vi "Turbulence_3.1_FullAuto.vi"() -> ()   [LabVIEW 2018]
uses:
  <instrlib>/Quantum Composers 9000 Series 2.08/Quantum Composers 9000 Series.lvlib
  <userlib>/LightField Add-in and Automation SDK/Samples/LabVIEW Automation/lightfield-automation-labview/LightField Automation.lvclass
  <instrlib>/Mercury iXX/Mercury iXX.lvlib
  <instrlib>/Mercury iXX/Public/Libraries/Temperature/Signals/Read/Temperature (Read).vi
  <instrlib>/Mercury iXX/Public/Libraries/Temperature.lvlib
  <instrlib>/Mercury iXX/Public/Libraries/Temperature/Open/Open Temperature Device.vi
  <instrlib>/Mercury iXX/Public/Controls/Comms Transport Layer.ctl
  <instrlib>/Keithley 2600 Series/Keithley 2600 Series.lvlib
  <instrlib>/Keithley 2600 Series/Public/Channel.ctl
  <vilib>/DAQmx/read.llb/DAQmx Read (Counter DBL 1Chan 1Samp).vi
  <instrlib>/Mercury iXX/Public/Libraries/System/Read/Catalogue (Read).vi
  <instrlib>/Mercury iXX/Public/Libraries/System.lvlib
  <instrlib>/Mercury iXX/Public/Libraries/System/Open/Open System.vi
panel:
  in  "Extra Waits":i32
  in  "Error":bool
  in  "3He Check":bool
  out "MFC Error Out":errorcluster
  out "Lakeshore218 Error":errorcluster
  in  "File Exists":bool
  out "Log":refnum<file>
  in  "Motor free":bool
  in  "RESTART":bool
  out "time string":string
  out "Timestamp":string
  out "Log Error":errorcluster
  in  "CLOSE":bool
  in  "RECORD":bool
  in  "Turbulence":T1(tab)
  in  "FROM FILE":bool
  in  "Script File":path
  in  "# Frames":i32=1000 min=0 step=1
  in  "New Background Movie":bool
  in  "On CCD Acc.":i32=3 min=0 step=1
  in  "Cycle time\n(ms)":i32=3 min=0 step=1
  out "High Level\n(Ohms)":dbl format="%.1f"
  out "Low Level\n(Ohms)":dbl format="%.1f"
  in  "New Background Frame":bool
  out "Rate (Hz)":dbl
  out "Incident":dbl
  in  "BIN":u16(ring)=2 items=["1x1", "2x2", "4x4"]
  in  "MODE":u16(ring) items=["Normal", "DIF"]
  in  "Enable":bool
  out "Rate (Hz)":dbl
  out "Detected":dbl
  in  "Script\nEnd":u32=1 step=1
  in  "Sample Space Pump":bool
  in  "Siphon Pump":bool
  in  "Neutron Shutter":bool
  in  "Manual Script Entry (0)":string
  in  "READY":bool
  out "Power (mW)":dbl format="%_3f"
  out "Tank Pressure 2 (Torr)":string="0.0"
  in  "LIGHTFIELD":bool
  in  "SCRIPTING":bool
  in  "Top Coil":bool
  out "Tank Pressure 1 (Torr)":string="0.0"
  out "Cell (K)":dbl format="%.3f"
  out "Cryostat (K)":dbl format="%.3f"
  in  "Data Interval (s)":dbl=0.5 min=0.4 max=10.0 step=0.05
  in  "RUN/STOP":bool
  in  "Bottom Coil":bool
  in  "Bottom Coil (mA)":dbl min=-1000.0 max=1000.0 step=1e-05
  in  "Top Coil (mA)":dbl min=-1000.0 max=1000.0 step=1e-05
  in  "Percent Open":i32 min=0 max=100 step=5
  in  "COOLDOWN":bool
  in  "Script\n#":i32 step=1
  in  "Kill Switch":bool
  in  "DATA":bool
  out "Scripting Error":T2
  in  "Shutter Mode":u16(ring)=1 items=["Manual"=1, "XGate"=5]
  in  "Time (s)":i32=120 min=1 max=300 step=1
  in  "REFILL":bool
  in  "AUTOFILL":bool
  in  "LL (Ohms)":dbl=900.0 min=750.0 max=15000.0 step=1.0
  in  "HL (Ohms)":dbl=900.0 min=750.0 max=15000.0 step=1.0
  in  "Fill":bool
  in  "Tare":bool
  out "Actual 3He\nTank Pressure":dbl min=0.0 max=100.0 step=5.0 format="%#.1g"
  out "Desired V2\nPressure (3He)":dbl min=0.0 max=100.0 step=5.0 format="%#.1f"
  in  "Desired Tank\nPressure (3He)":dbl min=0.0 max=100.0 step=0.01 format="%#.2f"
  in  "Log Pressure":bool
  out "4He Pressure (Torr)":string="-0.1"
  out "3He Pressure (Torr)":string="1"
  in  "Fill Time (s)":u32=10
  out "Temperature Error":errorcluster={"status"=TRUE, "code"=-1073807339, "source"="VISA Read in Mercury iXX.lvlib:Query (Dynamic).vit->Mercury iXX.lvlib:Query (Low Level).vi:10049->Mercury iXX.lvlib:Query.vi:3960048->Mercury iXX.lvlib:Read (Str).vi:5300004->Mercury iXX.lvlib:System.lvlib:Catalogue (Read).vi->Turbulence.vi"}
  out "File I/O Error":errorcluster
  out "4He Gauge Error":errorcluster={"status"=TRUE, "code"=-1073807343, "source"="VISA Open in Turbulence.vi"}
  out "Heater Error":errorcluster={"status"=FALSE, "code"=1073676293, "source"="VISA Read in Keithley 2600 Series.lvlib:Print Number.vi->Keithley 2600 Series.lvlib:Measure.vi->Turbulence.vi"}
  out "Pulse Generator Error":errorcluster
  out "3He Gauge Error":errorcluster={"status"=FALSE, "code"=1073676293, "source"="VISA Read in 3HeClose.vi->Turbulence.vi"}
  out "Relay Errror":errorcluster
  out "Zaber Motor Error":errorcluster
  out "LightField Error":errorcluster
  out "Shutter Error":errorcluster
  # "Camera Controls"
  # "Temperature Readout"
  # "Pressure Readout"
  # "Neutron Counts"
  # "Automation"
  # "Heater Controls"
  # "Relay Controls"
  # "Needle Valve Control"
  # "Neutron Shutter"
  # "Optical Shutter"
  # "Siphon Pump"
  # "Laser Power Meter"
  # "Sample Space\nPump"
  # "V1 = 4075 mL"
  # "V2 = 15.5 mL"
  # "V3 = 78.8 mL"
  # "Quartz\nCell"
  # "4"
  # "3psi relief"
  # "MFC"
  # "V1"
  # "4L Tank"
  # "Turbo Pump"
  # "V2"
  # "V3"
  # "3"
  # "10psi relief"
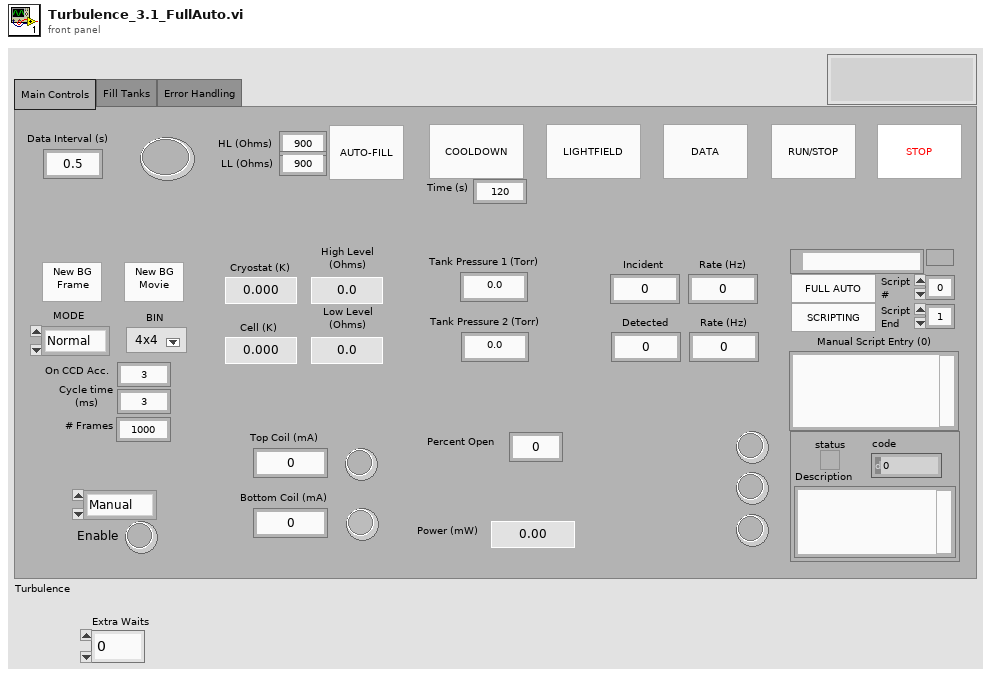
[diagram p1: front panel]
types:
  T1 = enum32{"Main Controls", "Fill Tanks", "Error Handling"}
  T2 = cluster{"status":bool, "code":i32, "Description":string}
  T3 = typedef "Mercury iXX.lvlib/Comms Transport Layer.ctl" = enum16{"Ethernet TCP/IP", "USB", "ISOBus - RS-232", "GPIB"}
  T4 = typedef "Mercury iXX.lvlib/Mercury Reference.ctl" = cluster{"Comms":refnum<visa-resource-name>, "Device ID":string[], "Comms Layer":T3, "Command":string, "Query reference":T5}
  T5 = typedef "Mercury iXX.lvlib/Query Dynamic Reference.ctl" = refnum<vi>
  T6 = enum32{"Current", "Voltage", "IV", "Resistance", "Power"}
  T7 = typedef "Keithley 2600 Series.lvlib/Channel.ctl" = enum32{"Channel A", "Channel B"}
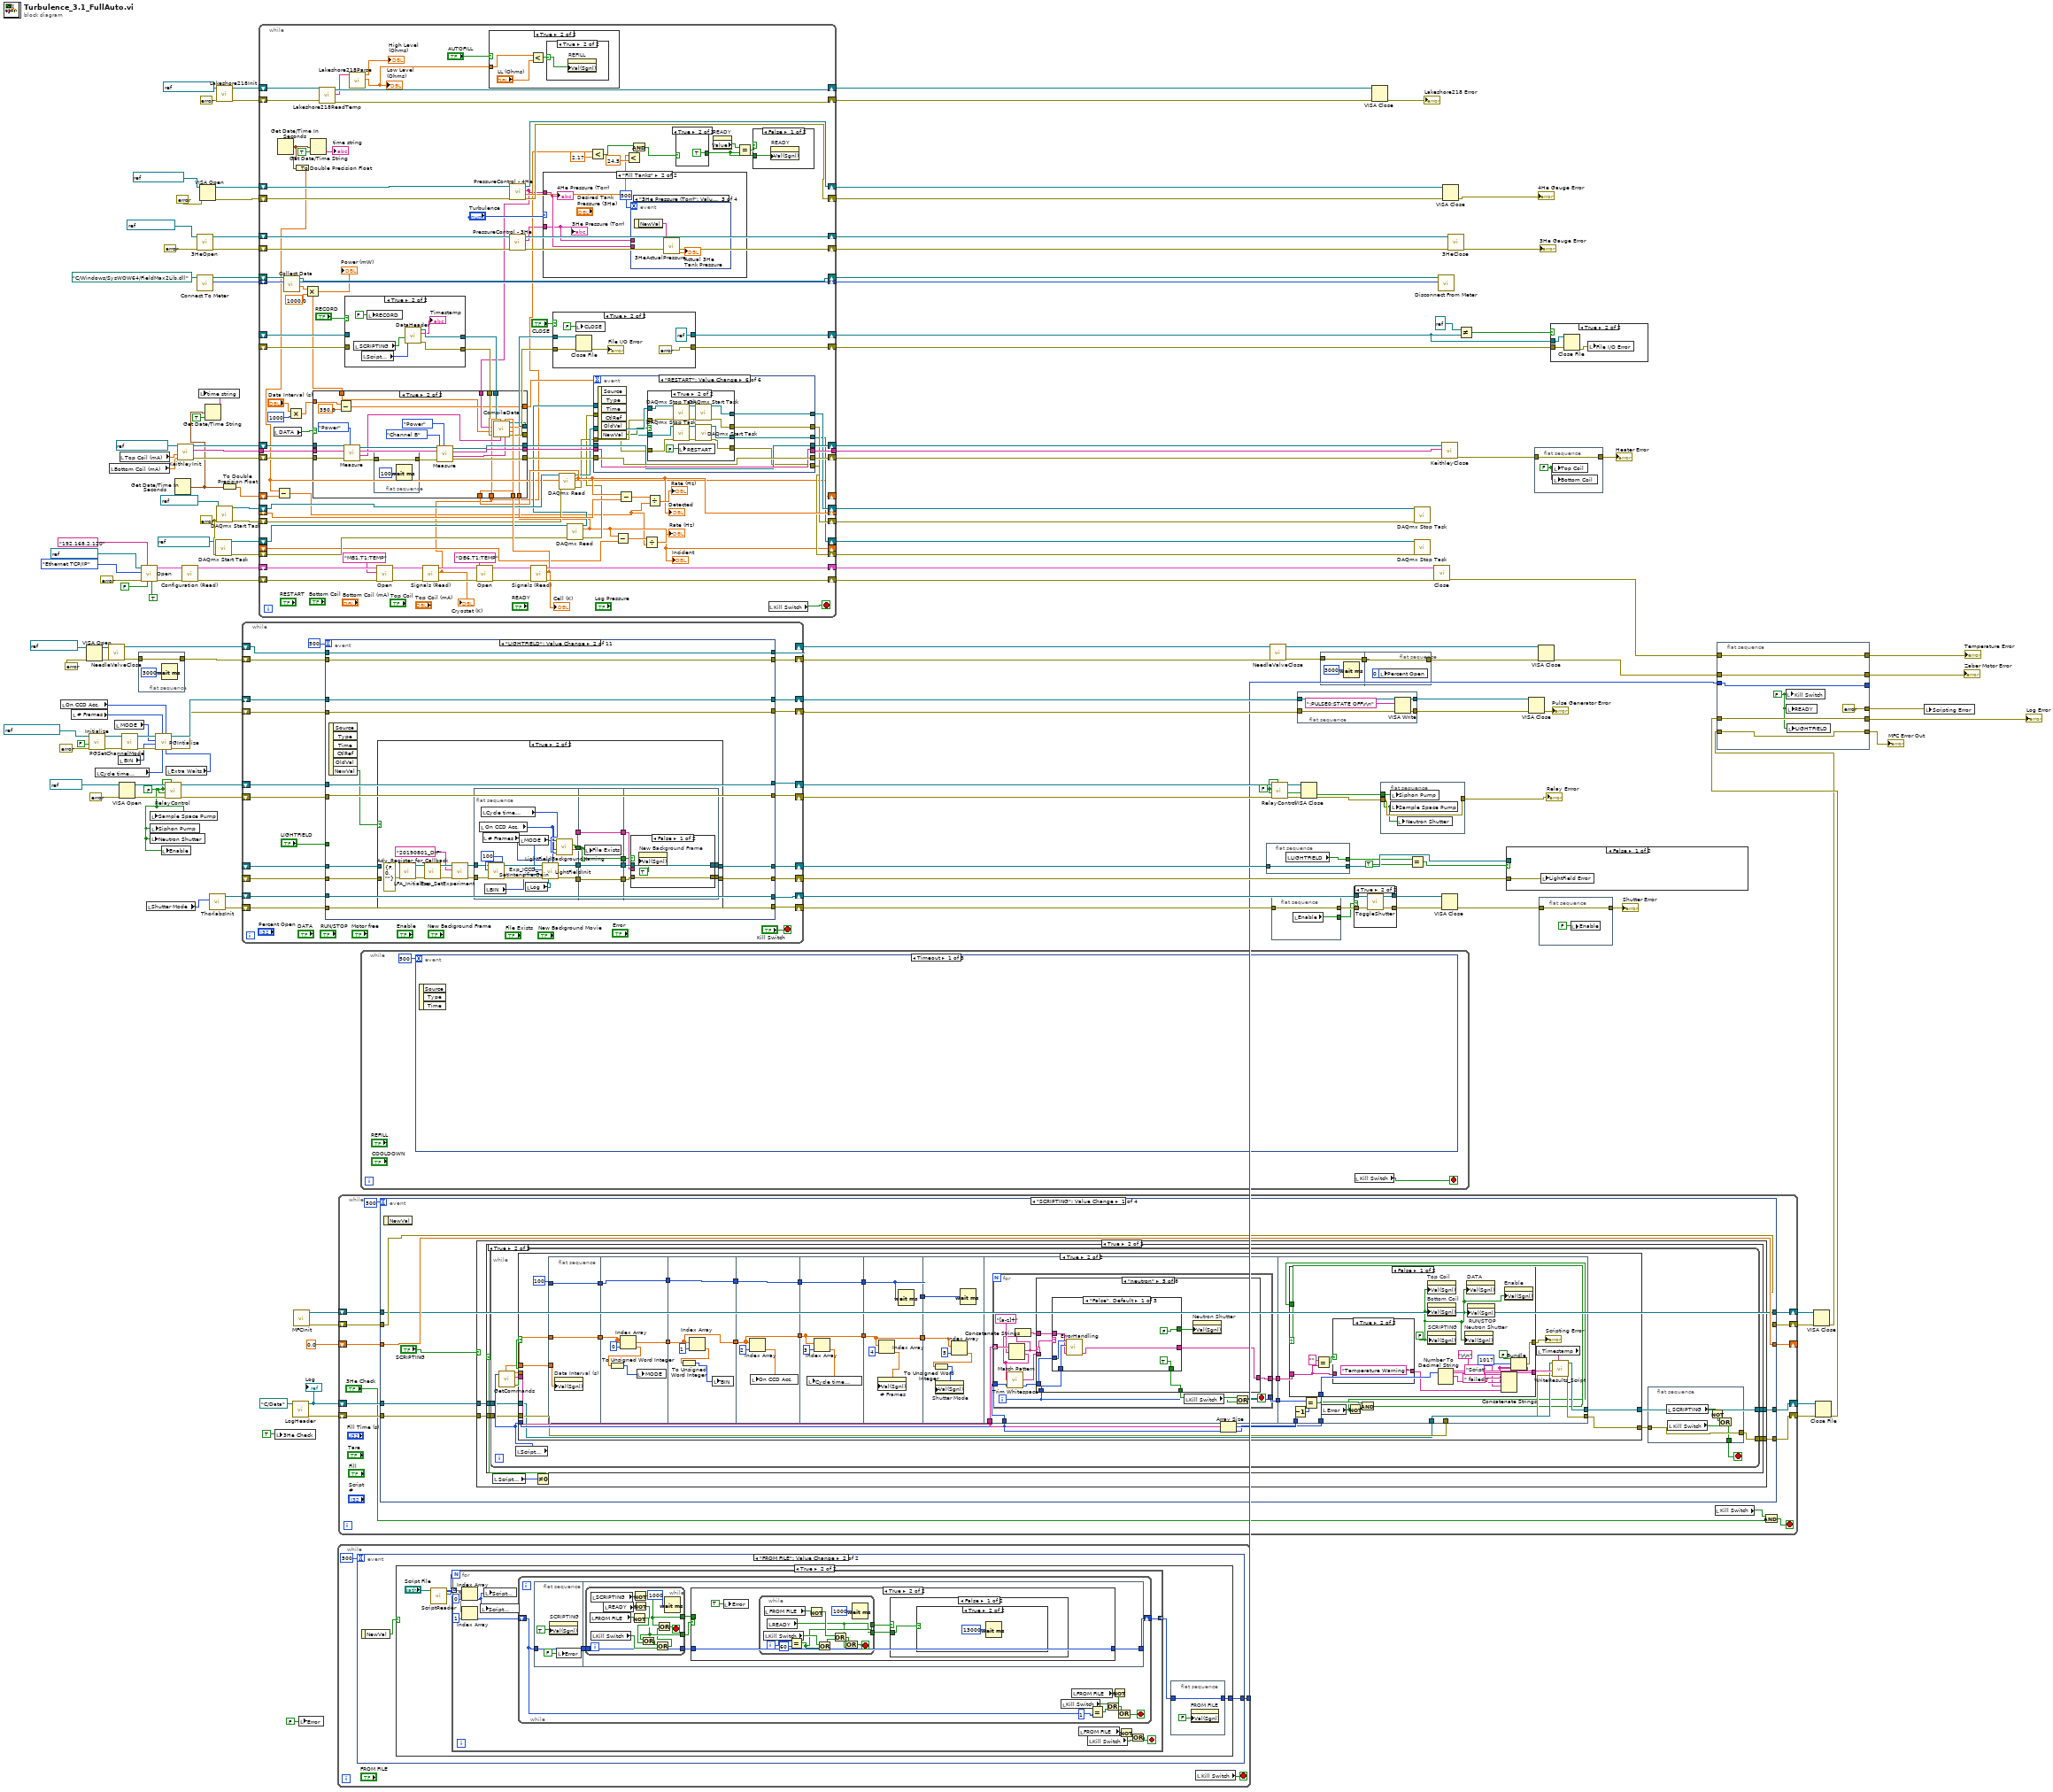
[diagram p0: block diagram]
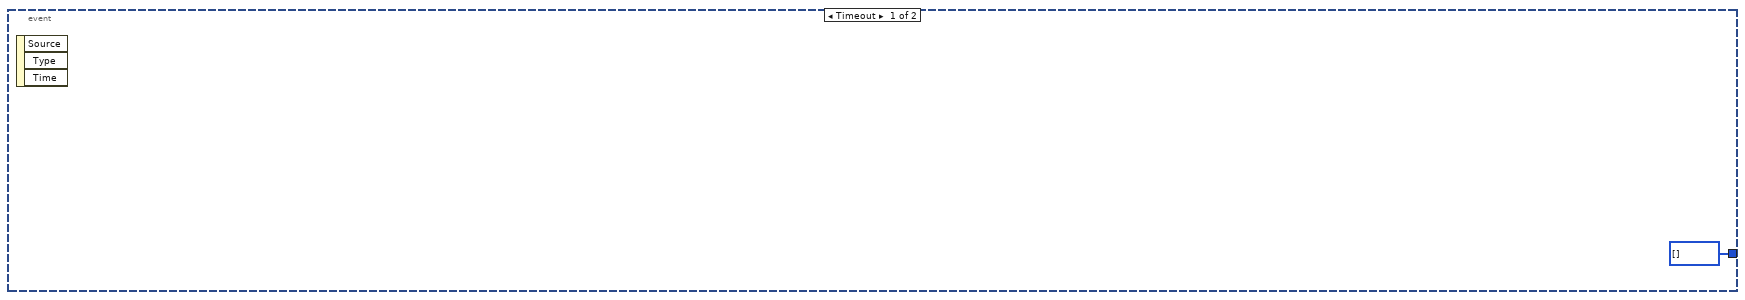
[diagram p2: hidden frame]
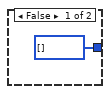
[diagram p3: hidden frame]
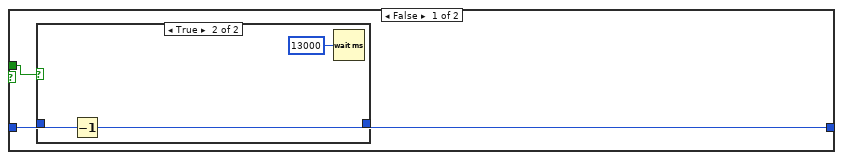
[diagram p4: hidden frame]
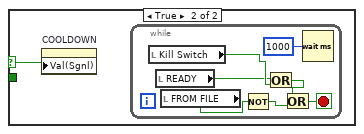
[diagram p7: hidden frame]
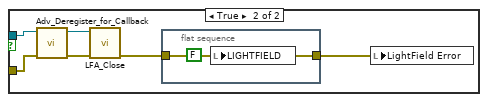
[diagram p9: hidden frame]
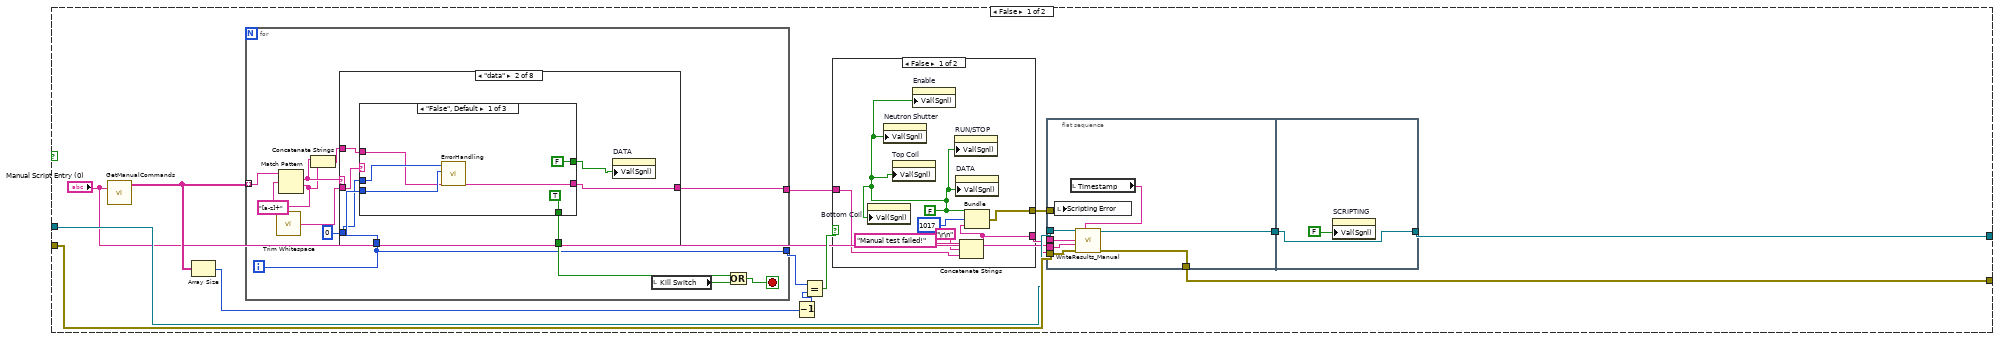
[diagram p11: hidden frame]
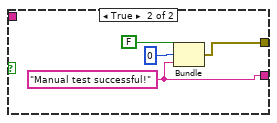
[diagram p12: hidden frame]
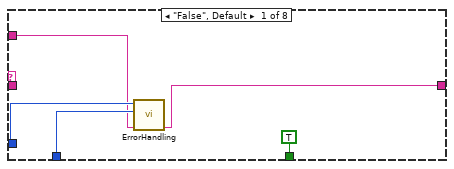
[diagram p13: hidden frame]
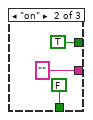
[diagram p14: hidden frame]
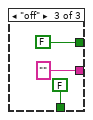
[diagram p15: hidden frame]
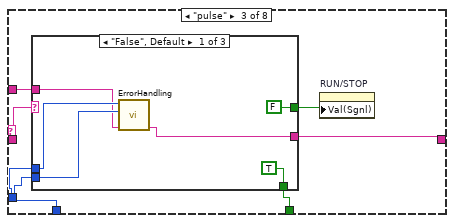
[diagram p16: hidden frame]
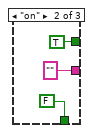
[diagram p17: hidden frame]
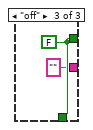
[diagram p18: hidden frame]
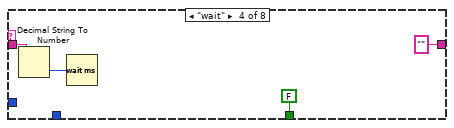
[diagram p19: hidden frame]
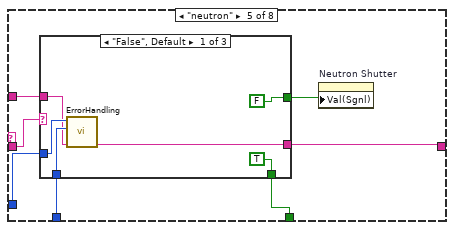
[diagram p20: hidden frame]
diagram:
  w42 = errorcluster {"status"=FALSE, "code"=0, "source"=""} ("error in")
  w79 = FALSE ("Siphon Pump")
  w64 = FALSE ("Siphon Pump")
  n1 = local read "On CCD Acc."() -> (w53:i32)
  n2 = local read "# Frames"() -> (w52:i32)
  n3 = VISA Open(error in (no error)=errorcluster {"status"=FALSE, "code"=0, "source"=""}, VISA resource name=refnum<visa-resource-name> "ZaberMotor") -> (VISA resource name=w59:refnum<visa-resource-name>, error out=w60:errorcluster)  [unwired: 3 in]
  n4 = call <instrlib>:"Initialize.vi"("error in (no error)"=errorcluster {"status"=FALSE, "code"=0, "source"=""}, "Reset? (T: Yes)"=FALSE, "VISA resource name"=refnum<visa-resource-name> "PulseGenerator" ("Pulse generater (COM3)")) -> ("error out"=w71:errorcluster, "VISA resource name out"=w69:refnum<visa-resource-name>)  [unwired: 7 in]
  n5 = local read "Cycle time\n(ms)"() -> (w13:i32)
  n6 = call "NeedleValveClose.vi"("error in (no error)"=w60, "VISA resource name"=w59) -> ("error out"=w61:errorcluster, "VISA resource name out"=w101:refnum<visa-resource-name>)  [unwired: 8 in]
  n7 = local read "Bottom Coil (mA)"() -> (w113:dbl)
  n8 = local read "MODE"() -> (w50:u16)
  n9 = local read "BIN"() -> (w51:u16)
  n10 = VISA Open(error in (no error)=errorcluster {"status"=FALSE, "code"=0, "source"=""} ("error in (no error) 2"), VISA resource name=refnum<visa-resource-name> "Relays" ("Pressure Gauge")) -> (VISA resource name=w126:refnum<visa-resource-name>, error out=w128:errorcluster)  [unwired: 3 in]
  n11 = local read "Top Coil (mA)"() -> (w114:dbl)
  n12 = call "PGSetChannelMode.vi"("error in"=w71, "VISA resource name"=w69) -> ("error out"=w70:errorcluster, "VISA resource name out"=w68:refnum<visa-resource-name>)  [unwired: 8 in]
  n13 = flat-sequence {
    tunnel: w61 -> [w155]
    tunnel: [w155] -> w102
    frame #0 {
      n14 = Wait (ms)(milliseconds to wait=u32 3000) -> ()  [unwired: 1 out]
    }
  }
  n15 = call-poly <instrlib>:"Open.vi"("Clear Previous Connections (False)"=TRUE, "ID Query (True)"=FALSE, "IP Address"="192.168.2.120", "error in (no error)"=errorcluster {"status"=FALSE, "code"=0, "source"=""}, "Comms Layer"=Comms_Transport_Layer."Ethernet TCP/IP", "VISA resource name"=refnum<visa-resource-name> "MercuryiTC") -> ("error out"=w147:errorcluster, "Mercury Reference Out"=w148:T4)  [unwired: 1 in, 3 out]
  n16 = local read "Shutter Mode"() -> (w54:u16)
  n17 = local write "Sample Space Pump"(w64) -> ()
  n18 = local write "Neutron Shutter"(w64) -> ()
  n19 = local write "Siphon Pump"(w64) -> ()
  n20 = local write "Enable"(w64) -> ()
  n21 = call "RelayControl.vi"("Neutron Shutter"=w64, "Error In"=w128, "Sample Space Pump"=w64, "Siphon Pump"=w64, "Relay In"=w126) -> ("Error Out"=w127:errorcluster, "Relay Out"=w125:refnum<visa-resource-name>)  [unwired: 5 in]
  n22 = local read "Extra Waits"() -> (w1:i32)
  n23 = call "PGIntialize.vi"("Extra Waits"=w1, "On CCD Accumulations"=w53, "Cycle time\n(ms)"=w13, "Number of Frames"=w52, "error in"=w70, "BIN"=w51, "MODE"=w50, "VISA resource name"=w68) -> ("error out"=w152:errorcluster, "VISA resource name out"=w153:refnum<visa-resource-name>)  [unwired: 2 in]
  n24 = Get Date/Time In Seconds() -> (seconds since 1Jan1904=w21:timestamp)
  n25 = call "KeithleyInit.vi"("Bottom Coil (mA)"=w113, "Top Coil (mA)"=w114, "KeithleyVISA In"=refnum<visa-resource-name> "Keithley2614B" ("VISA resource name")) -> ("error out"=w117:errorcluster, "Node Out"=w118:string, "KeithleyVISA Out"=w116:refnum<visa-resource-name>)  [unwired: 6 in]
  n26 = call-poly <instrlib>:"Configuration (Read).vi"("error in"=w147, "Mercury Reference In"=w148) -> ("error out"=w143:errorcluster, "Mercury Reference Out"=w144:T4)  [unwired: 6 in, 2 out]
  n27 = call "Connect To Meter.vi"("Location of FieldMax2Lib.dll in"=path "C:/Windows/SysWOW64/FieldMax2Lib.dll") -> ("Meter ID out"=w87:i32, "Location of FieldMax2Lib.dll out"=w86:path)  [unwired: 6 in, 1 out]
  n28 = call "3HeOpen.vi"("error in (no error)"=errorcluster {"status"=FALSE, "code"=0, "source"=""} ("error in (no error) 2"), "VISA resource name"=refnum<visa-resource-name> "3HePressure" ("Pressure Gauge")) -> ("error out"=w130:errorcluster, "VISA resource name out"=w129:refnum<visa-resource-name>)  [unwired: 8 in]
  n29 = VISA Open(error in (no error)=errorcluster {"status"=FALSE, "code"=0, "source"=""} ("error in (no error) 2"), VISA resource name=refnum<visa-resource-name> "TankPressure" ("Pressure Gauge")) -> (VISA resource name=w140:refnum<visa-resource-name>, error out=w141:errorcluster)  [unwired: 3 in]
  n30 = Get Date/Time String(seconds (now)=w21, want seconds? (F)=TRUE) -> (time string=w22:string)  [unwired: 1 in, 1 out]
  n31 = local write "time string"(w22) -> ()
  n32 = call "ThorlabsInit.vi"("Shutter Mode"=w54) -> ("error out"=w65:errorcluster, "VISA resource name out"=w66:refnum<visa-resource-name>)  [unwired: 9 in]
  n33 = call <vilib>:"DAQmx Start Task.vi"("task/channels in"=refnum<k21> "IncidentBeam", "error in"=w42) -> ("task out"=w44:refnum<k21>, "error out"=w43:errorcluster)  [unwired: 12 in]
  n34 = call "Lakeshore218Init.vi"("error in (no error)"=errorcluster {"status"=FALSE, "code"=0, "source"=""}, "VISA resource name"=refnum<visa-resource-name> "Lakeshore218") -> ("error out"=w19:errorcluster, "VISA resource name out"=w18:refnum<visa-resource-name>)  [unwired: 8 in]
  n35 = call <vilib>:"DAQmx Start Task.vi"("task/channels in"=refnum<k21> "Detector", "error in"=w42) -> ("task out"=w47:refnum<k21>, "error out"=w46:errorcluster)  [unwired: 12 in]
  n36 = To Double Precision Float(number=w21) -> (double precision float=w24:dbl)
  n37 = while {
    shift-right: [w178] -> w31
    shift-left: _ -> [w176]
    shift-right: [w179] -> w38
    shift-left: _ -> [w177]
    shift-right: [w172] -> w95
    shift-left: w153 -> [w174]
    shift-right: [w173] -> w96
    shift-left: w152 -> [w175]
    shift-right: [w168] -> w100
    shift-left: w127 -> [w171]
    shift-right: [w169] -> w98
    shift-left: w125 -> [w170]
    shift-right: [w163] -> w131
    shift-left: w102 -> [w166]
    shift-right: [w164] -> w132
    shift-left: w101 -> [w165]
    shift-right: [w160] -> w34
    shift-left: w66 -> [w157]
    shift-right: [w159] -> w27
    shift-left: w65 -> [w158]
    stop <- "Kill Switch" stop-if-true
    n38 = event shown="[1] \"LIGHTFIELD\": Value Change" {
      selector: _ -> [_ _ _ _ _ _ _ _ _ _ _]
      dyn-events: _ -> [_ _ _ _ _ _ _ _ _ _ _]
      timeout: 500 -> [_ _ _ _ _ _ _ _ _ _ _]
      tunnel: w175 -> [w187 w196 w273 w319 w337 w386 w451 w470 w485 w508 w533]
      tunnel: w174 -> [w186 w195 w274 w320 w336 w387 w452 w469 w484 w507 w534]
      tunnel: w177 -> [w188 w199 w264 w311 w339 w390 w449 w473 w489 w499 w529]
      tunnel: w176 -> [w189 w200 w265 w312 w340 w391 w450 w474 w488 w500 w530]
      tunnel: [w188 w201 w263 w311 w339 w378 w449 w473 w489 w499 w529] -> w179
      tunnel: [w189 w202 w262 w312 w340 w370 w450 w474 w488 w500 w530] -> w178
      tunnel: [w187 w196 w276 w319 w337 w376 w451 w470 w485 w505 w533] -> w173
      tunnel: [w186 w195 w275 w320 w336 w383 w452 w469 w484 w506 w534] -> w172
      tunnel: w171 -> [w184 w197 w270 w317 w342 w385 w458 w472 w487 w501 w531]
      tunnel: w170 -> [w185 w198 w271 w318 w341 w384 w457 w471 w486 w502 w532]
      tunnel: [w185 w198 w271 w318 w341 w384 w454 w471 w486 w502 w532] -> w169
      tunnel: [w184 w197 w270 w317 w342 w385 w453 w472 w487 w501 w531] -> w168
      tunnel: w166 -> [w183 w194 w269 w321 w325 w389 w448 w468 w483 w503 w535]
      tunnel: w165 -> [w182 w193 w268 w322 w338 w388 w447 w467 w482 w504 w536]
      tunnel: [w182 w193 w268 w322 w335 w388 w447 w467 w482 w504 w536] -> w164
      tunnel: [w183 w194 w269 w321 w327 w389 w448 w468 w483 w503 w535] -> w163
      tunnel: "LIGHTFIELD" -> [_ _ w261 w316 _ w372 _ _ _ w495 _]
      tunnel: w157 -> [w180 w191 w267 w314 w333 w382 w445 w466 w493 w498 w528]
      tunnel: w158 -> [w181 w190 w266 w313 w332 w381 w444 w465 w492 w497 w527]
      tunnel: [w180 w191 w267 w314 w333 w382 w445 w463 w490 w498 w528] -> w160
      tunnel: [w181 w190 w266 w313 w332 w381 w444 w464 w491 w497 w527] -> w159
      event Timeout {
        n39 = event-data() -> ()  [unwired: 1 in, 3 out]
      }
      event "LIGHTFIELD": Value Change {
        n40 = event-data() -> ("NewVal"=w192:bool)  [unwired: 1 in, 5 out]
        n41 = case shown="True" w192 {
          tunnel: [refnum<class "LightField Automation.lvclass"> refnum ("LightField Automation out") w218] -> w202
          tunnel: [errorcluster {"status"=FALSE, "code"=0, "source"=""} ("error out") w217] -> w201
          tunnel: w200 -> [w206 _]
          tunnel: w199 -> [w205 _]
          frame False {
            n42 = call <userlib>:"Adv_Deregister_for_Callback.vi"("error in (no error)"=w205, "LightField Automation in"=w206) -> ("error out"=w208:errorcluster, "LightField Automation out"=w209:refnum<class "LightField Automation.lvclass">)  [unwired: 8 in]
            n43 = call <userlib>:"LFA_Close.vi"("error in (no error)"=w208, "LightField Automation in"=w209) -> ("error out"=→"LightField Error":errorcluster)  [unwired: 8 in, 1 out]
          }
          frame True {
            n44 = call <userlib>:"LFA_Initialize.vi"("error in (no error)"=errorcluster {"status"=FALSE, "code"=0, "source"=""}) -> ("error out"=w227:errorcluster, "LightField Automation out"=w226:refnum<class "LightField Automation.lvclass">)  [unwired: 9 in]
            n45 = call <userlib>:"Adv_Register_for_Callback.vi"("error in (no error)"=w227, "LightField Automation in"=w226) -> ("error out"=w225:errorcluster, "LightField Automation out"=w224:refnum<class "LightField Automation.lvclass">)  [unwired: 8 in]
            n46 = call <userlib>:"Exp_SetExperiment.vi"("error in (no error)"=w225, "ExperimentName"="20190801_DIF", "LightField Automation in"=w224) -> ("error out"=w211:errorcluster, "LightField Automation out"=w210:refnum<class "LightField Automation.lvclass">)  [unwired: 7 in]
            n47 = flat-sequence {
              tunnel: [w238] -> w215
              tunnel: [w236] -> w214
              tunnel: [w235] -> w213
              tunnel: [w239] -> w212
              tunnel: w211 -> [w242]
              tunnel: w210 -> [w240]
              tunnel: [w246] -> w221
              tunnel: [w245] -> w220
              tunnel: [w244] -> w219
              tunnel: [w243] -> w216
              tunnel: w215 -> [w243]
              tunnel: w214 -> [w246]
              tunnel: w213 -> [w245]
              tunnel: w212 -> [w244]
              tunnel: w221 -> [w251]
              tunnel: w220 -> [w252]
              tunnel: w219 -> [w250]
              tunnel: [w249] -> w218
              tunnel: [w248] -> w217
              tunnel: w216 -> [w247]
              frame #0 {
                n48 = local read "On CCD Acc."() -> (w228:i32)
                n49 = local read "Cycle time\n(ms)"() -> (w237:i32)
                n50 = local read "# Frames"() -> (w229:i32)
                n51 = local read "BIN"() -> (w231:u16)
                n52 = call <userlib>:"Exp_ICCD_SetIntensifierGain.vi"("error in (no error)"=w242, "Intensifier Gain"=100, "LightField Automation in"=w240) -> ("error out"=w233:errorcluster, "LightField Automation out"=w234:refnum<class "LightField Automation.lvclass">)  [unwired: 7 in]
                n53 = local read "MODE"() -> (w230:u16)
                n54 = local read "Log"() -> (w232:refnum<file>)
                n55 = call "LightFieldInit.vi"("On CCD Accumulations"=w228, "File Path"=w232, "Number of Frames"=w229, "error in"=w233, "BIN"=w231, "MODE"=w230, "LightField Automation in"=w234) -> ("error out"=w236:errorcluster, "LightField Automation out"=w235:refnum<class "LightField Automation.lvclass">)  [unwired: 3 in]
                n56 = call "LightFieldBackgroundNaming.vi"("Cycle time\n(ms)"=w237, "On CCD Acc."=w228, "MODE"=w230) -> ("FilePath"=w239:string, "Exists"=w238:bool)  [unwired: 6 in, 1 out]
              }
              frame #1 {
                n57 = local write "File Exists"(w243) -> ()
              }
              frame #2 {
                n58 = case shown="False" w247 {
                  tunnel: w252 -> [w255 w260]
                  tunnel: w251 -> [w254 w259]
                  tunnel: w250 -> [_ w258]
                  tunnel: [w255 w257] -> w249
                  tunnel: [w254 w256] -> w248
                  frame False {
                    n59 = property on="New Background Frame" class="Bool (strict)"("Val(Sgnl)"=TRUE ("Value (Signaling)")) -> ()  [unwired: 2 in, 2 out]
                  }
                  frame True {
                    n60 = call "LightFieldChangeBackground.vi"("error in"=w259, "FilePath"=w258, "LightField Automation in"=w260) -> ("error out"=w256:errorcluster, "LightField Automation out"=w257:refnum<class "LightField Automation.lvclass">)  [unwired: 7 in]
                  }
                }
              }
            }
          }
        }
      }
      event "RUN/STOP": Value Change {
        n61 = event-data() -> ("NewVal"=w272:bool)  [unwired: 1 in, 5 out]
        n62 = case shown="True" w272 {
          tunnel: [w280 w293] -> w276
          tunnel: [w281 w292] -> w275
          tunnel: w274 -> [w282 w291]
          tunnel: w273 -> [w283 w290]
          tunnel: w265 -> [w278 w288]
          tunnel: w264 -> [w277 w287]
          tunnel: [w277 w286] -> w263
          tunnel: [w278 w285] -> w262
          tunnel: w261 -> [_ w284]
          frame False {
            n63 = VISA Write(VISA resource name=w282, write buffer=":PULSE0:STATE OFF\r\n" ("format string"), error in (no error)=w283) -> (VISA resource name out=w281:refnum<visa-resource-name>, error out=w280:errorcluster)  [unwired: 1 out]
          }
          frame True {
            n64 = case shown="True" w284 {
              tunnel: w287 -> [w294 w306]
              tunnel: w288 -> [w295 w304]
              tunnel: [w295 w308] -> w285
              tunnel: [w294 w307] -> w286
              frame False {
              }
              frame True {
                n65 = local read "New Background Movie"() -> (w298:bool)
                n66 = local read "Cycle time\n(ms)"() -> (w296:i32)
                n67 = local read "On CCD Acc."() -> (w297:i32)
                n68 = local read "MODE"() -> (w301:u16)
                n69 = local read "SCRIPTING"() -> (w299:bool)
                n70 = local read "BIN"() -> (w302:u16)
                n71 = case shown="True" w299 {
                  tunnel: [-1 ("Script\n#") w310] -> w300
                  frame False {
                  }
                  frame True {
                    n72 = local read "Script\n#"() -> (w310:i32)
                  }
                }
                n73 = call "LightFieldFileNaming.vi"("Cycle time\n(ms)"=w296, "On CCD Acc."=w297, "Script#"=w300, "BG"=w298, "error in"=w306, "BIN"=w302, "MODE"=w301, "LightField Automation in"=w304) -> ("error out"=w305:errorcluster, "LightField Automation out"=w303:refnum<class "LightField Automation.lvclass">)  [unwired: 2 in]
                n74 = call <instrlib>:"LFA_Acquire.vi"("error in (no error)"=w305, "LightField Automation in"=w303) -> ("error out"=w307:errorcluster, "LightField Automation out"=w308:refnum<class "LightField Automation.lvclass">)  [unwired: 8 in]
              }
            }
            n75 = VISA Write(VISA resource name=w291, write buffer=":PULSE0:STATE ON\r\n" ("format string"), error in (no error)=w290) -> (VISA resource name out=w292:refnum<visa-resource-name>, error out=w293:errorcluster)  [unwired: 1 out]
          }
        }
      }
      event "DATA": Value Change {
        n76 = event-data() -> ("NewVal"=w315:bool)  [unwired: 1 in, 5 out]
        n77 = case shown="False" w315 {
          tunnel: w316 -> [_ _]
          frame False {
            n78 = local write "CLOSE"(TRUE ("CLOSE")) -> ()
          }
          frame True {
            n79 = local write "RECORD"(TRUE ("RECORD")) -> ()
          }
        }
      }
      event "Percent Open": Value Change {
        n80 = event-data() -> ("OldVal"=w334:i32, "NewVal"=w343:i32)  [unwired: 1 in, 4 out]
        n81 = flat-sequence {
          tunnel: w325 -> [w345]
          tunnel: [w345] -> w326
          frame #0 {
            n82 = property on="Motor free" class="Bool (strict)"("Val(Sgnl)"=FALSE ("Value (Signaling)")) -> ()  [unwired: 2 in, 2 out]
          }
        }
        n83 = Subtract(x=w343, y=w334) -> (x-y=w329:i32)
        n84 = Greater Than 0?(x=w329) -> (x > 0?=w330:bool)
        n85 = Equal To 0?(x=w343) -> (x = 0?=w331:bool)
        n86 = case shown="False" w331 {
          tunnel: w338 -> [w351 w367]
          tunnel: w326 -> [w352 w366]
          tunnel: [w350 w365] -> w335
          tunnel: [w349 w364] -> w328
          tunnel: w330 -> [w353 _]
          tunnel: w329 -> [w348 _]
          frame False {
            n87 = case shown="True" w353 {
              tunnel: w352 -> [w357 w363]
              tunnel: w351 -> [w358 w362]
              tunnel: [w356 w361] -> w350
              tunnel: [w355 w360] -> w349
              tunnel: w348 -> [w354 w359]
              frame False {
                n88 = call "NeedleValveClose - Encoder.vi"("error in (no error)"=w357, "Percent Difference"=w354, "VISA resource name"=w358) -> ("error out"=w355:errorcluster, "VISA resource name out"=w356:refnum<visa-resource-name>)  [unwired: 7 in]
              }
              frame True {
                n89 = call "NeedleValveOpen - Encoder.vi"("error in (no error)"=w363, "Percent Difference"=w359, "VISA resource name"=w362) -> ("error out"=w360:errorcluster, "VISA resource name out"=w361:refnum<visa-resource-name>)  [unwired: 7 in]
              }
            }
          }
          frame True {
            n90 = call "NeedleValveClose.vi"("error in (no error)"=w366, "VISA resource name"=w367) -> ("error out"=w364:errorcluster, "VISA resource name out"=w365:refnum<visa-resource-name>)  [unwired: 8 in]
          }
        }
        n91 = flat-sequence {
          tunnel: w328 -> [w347]
          tunnel: [w347] -> w327
          frame #0 {
            n92 = property on="Motor free" class="Bool (strict)"("Val(Sgnl)"=TRUE ("Value (Signaling)")) -> ()  [unwired: 2 in, 2 out]
          }
        }
      }
      event "Cycle time\n(ms)", "# Frames", "MODE", "BIN", "On CCD Acc.", "Extra Waits": Value Change {
        n93 = event-data() -> ()  [unwired: 1 in, 1 out]
        n94 = case shown="True" w372 {
          tunnel: w391 -> [w432 w440]
          tunnel: w390 -> [w433 w441]
          tunnel: [w432 w439] -> w371
          tunnel: [w433 w438] -> w379
          tunnel: "On CCD Acc." -> [_ w436]
          tunnel: "# Frames" -> [_ w437]
          tunnel: "BIN" -> [_ w435]
          tunnel: "MODE" -> [_ w434]
          frame False {
          }
          frame True {
            n95 = call "LightFieldParams.vi"("On CCD Accumulations"=w436, "Number of Frames"=w437, "error in"=w441, "BIN"=w435, "MODE"=w434, "LightField Automation in"=w440) -> ("error out"=w438:errorcluster, "LightField Automation out"=w439:refnum<class "LightField Automation.lvclass">)  [unwired: 4 in]
          }
        }
        n96 = call "PGIntialize.vi"("Extra Waits"="Extra Waits", "On CCD Accumulations"="On CCD Acc.", "Cycle time\n(ms)"="Cycle time\n(ms)", "Number of Frames"="# Frames", "error in"=w386, "BIN"="BIN", "MODE"="MODE", "VISA resource name"=w387) -> ("error out"=w377:errorcluster, "VISA resource name out"=w383:refnum<visa-resource-name>)  [unwired: 2 in]
        n97 = case shown="True" w372 {
          tunnel: w379 -> [w394 w404]
          tunnel: [w394 w403] -> w378
          tunnel: w377 -> [w393 w402]
          tunnel: [w393 w401] -> w376
          tunnel: "On CCD Acc." -> [_ w400]
          tunnel: "BIN" -> [_ w399]
          tunnel: "MODE" -> [_ w398]
          tunnel: w371 -> [w392 w397]
          tunnel: [w392 w396] -> w370
          tunnel: "Cycle time\n(ms)" -> [_ w395]
          frame False {
          }
          frame True {
            n98 = flat-sequence {
              tunnel: w404 -> [w408]
              tunnel: [w407] -> w403
              tunnel: w402 -> [w416]
              tunnel: [w416] -> w401
              tunnel: w400 -> [w415]
              tunnel: w399 -> [w414]
              tunnel: w398 -> [w413]
              tunnel: w397 -> [w409]
              tunnel: [w406] -> w396
              tunnel: w395 -> [w405]
              frame #0 {
                n99 = call "LightFieldBackgroundNaming.vi"("Cycle time\n(ms)"=w405, "On CCD Acc."=w415, "BIN"=w414, "MODE"=w413) -> ("FilePath"=w410:string, "Exists"=w412:bool)  [unwired: 5 in, 1 out]
                n100 = flat-sequence {
                  tunnel: w412 -> [w417]
                  tunnel: [w417] -> w411
                  tunnel: w411 -> [w423]
                  tunnel: w410 -> [w422]
                  tunnel: w409 -> [w421]
                  tunnel: w408 -> [w420]
                  tunnel: [w419] -> w407
                  tunnel: [w418] -> w406
                  frame #0 {
                    n101 = local write "File Exists"(w417) -> ()
                  }
                  frame #1 {
                    n102 = case shown="True" w423 {
                      tunnel: w422 -> [_ w431]
                      tunnel: w421 -> [w425 w430]
                      tunnel: w420 -> [w424 w429]
                      tunnel: [w424 w428] -> w419
                      tunnel: [w425 w427] -> w418
                      frame False {
                        n103 = property on="New Background Frame" class="Bool (strict)"("Val(Sgnl)"=TRUE ("Value (Signaling)")) -> ()  [unwired: 2 in, 2 out]
                      }
                      frame True {
                        n104 = call "LightFieldChangeBackground.vi"("error in"=w429, "FilePath"=w431, "LightField Automation in"=w430) -> ("error out"=w428:errorcluster, "LightField Automation out"=w427:refnum<class "LightField Automation.lvclass">)  [unwired: 7 in]
                      }
                    }
                  }
                }
              }
            }
          }
        }
      }
      event "Siphon Pump", "Sample Space Pump", "Neutron Shutter": Value Change {
        n105 = event-data() -> ("CtlRef"=w442:refnum<vi>)  [unwired: 1 in]
        n106 = property class="Bool (strict)"(reference=w442) -> ("Label.Text"=w443:string)  [unwired: 1 in, 2 out]
        n107 = call "RelayControl.vi"("Neutron Shutter"="Neutron Shutter", "Error In"=w458, "Sample Space Pump"="Sample Space Pump", "Siphon Pump"="Siphon Pump", "Relay In"=w457) -> ("Error Out"=w453:errorcluster, "Relay Out"=w454:refnum<visa-resource-name>)  [unwired: 5 in]
        n108 = case shown="\"Neutron Shutter\"" w443 {
          frame "0", Default {
          }
          frame "Neutron Shutter" {
            n109 = property on="RESTART" class="Bool (strict)"("Val(Sgnl)"=TRUE ("RESTART")) -> ()  [unwired: 2 in, 2 out]
          }
        }
      }
      event "Enable": Value Change {
        n110 = event-data() -> ("OldVal"=w461:bool, "NewVal"=w462:bool)  [unwired: 1 in, 4 out]
        n111 = Not Equal?(x=w461, y=w462) -> (x != y?=w460:bool)
        n112 = case shown="True" w460 {
          tunnel: w466 -> [w476 w480]
          tunnel: w465 -> [w475 w479]
          tunnel: [w475 w478] -> w464
          tunnel: [w476 w477] -> w463
          frame False {
          }
          frame True {
            n113 = call "ToggleShutter.vi"("error in"=w479, "VISA resource name"=w480) -> ("error out"=w478:errorcluster, "VISA resource name out"=w477:refnum<visa-resource-name>)  [unwired: 8 in]
          }
        }
      }
      event "Shutter Mode": Value Change {
        n114 = event-data() -> ()  [unwired: 1 in, 6 out]
        n115 = call "ThorlabsMode.vi"("error in"=w492, "Mode"="Shutter Mode", "VISA resource name"=w493) -> ("error out"=w491:errorcluster, "VISA resource name out"=w490:refnum<visa-resource-name>)  [unwired: 7 in]
      }
      event "New Background Frame": Value Change {
        n116 = event-data() -> ("NewVal"=w496:bool)  [unwired: 1 in]
        n117 = And(x=w496, y=w495) -> (x .and. y?=w494:bool)
        n118 = case shown="True" w494 {
          tunnel: w508 -> [w509 w522]
          tunnel: w507 -> [w510 w523]
          tunnel: [w510 w520] -> w506
          tunnel: [w509 w514] -> w505
          frame False {
          }
          frame True {
            n119 = local read "Cycle time\n(ms)"() -> (w512:i32)
            n120 = local read "On CCD Acc."() -> (w521:i32)
            n121 = local read "MODE"() -> (w517:u16)
            n122 = local read "File Exists"() -> (w513:bool)
            n123 = local read "Extra Waits"() -> (w511:i32)
            n124 = local read "BIN"() -> (w516:u16)
            n125 = call "LightFieldAcquireBackground.vi"("Cycle time\n(ms)"=w512, "File Exists"=w513, "On CCD Acc."=w521, "error in"=w522, "BIN"=w516, "MODE"=w517, "VISA resource name"=w523) -> ("error out"=w519:errorcluster, "VISA resource name out"=w518:refnum<visa-resource-name>)  [unwired: 3 in]
            n126 = call "PGResetCameraWait.vi"("Extra Waits"=w511, "Cycle time\n(ms)"=w512, "error in"=w519, "BIN"=w516, "MODE"=w517, "VISA resource name"=w518) -> ("error out"=w515:errorcluster, "VISA resource name out"=w520:refnum<visa-resource-name>)  [unwired: 4 in]
            n127 = flat-sequence {
              tunnel: w515 -> [w525]
              tunnel: [w525] -> w514
              frame #0 {
                n128 = local write "New Background Frame"(FALSE ("New Background")) -> ()
                n129 = local write "File Exists"(TRUE ("File Exists")) -> ()
              }
            }
          }
        }
      }
      event "New Background Movie": Value Change {
        n130 = event-data() -> ("NewVal"=w537:bool)  [unwired: 1 in]
        n131 = case shown="True" w537 {
          frame False {
          }
          frame True {
            n132 = flat-sequence {
              tunnel: [w557] -> w548
              tunnel: w547 -> [w556]
              tunnel: [w556] -> w546
              tunnel: [w555] -> w545
              tunnel: w542 -> [w554]
              tunnel: [w554] -> w541
              tunnel: w548 -> [w561]
              tunnel: w546 -> [w562]
              tunnel: w545 -> [w559]
              tunnel: [w561] -> w544
              tunnel: [w559] -> w543
              tunnel: w541 -> [w558]
              tunnel: [w558] -> w540
              tunnel: w544 -> [w568]
              tunnel: w543 -> [w567]
              tunnel: w540 -> [w565]
              tunnel: [w568] -> w539
              tunnel: [w567] -> w538
              tunnel: w539 -> [w569]
              tunnel: w538 -> [w570]
              frame #0 {
                n133 = local read "Manual Script Entry (0)"() -> (w557:string)
                n134 = local read "Script\n#"() -> (w555:i32)
                n135 = Wait (ms)(milliseconds to wait=u32 15) -> ()  [unwired: 1 out]
              }
              frame #1 {
                n136 = local write "Manual Script Entry (0)"(w562) -> ()
                n137 = local write "Script\n#"(0 ("Script\n#")) -> ()
              }
              frame #2 {
                n138 = Add(x=w565, y=500) -> (x+y=w563:i32)
                n139 = property on="SCRIPTING" class="Bool (strict)"("Val(Sgnl)"=TRUE ("Value (Signaling)")) -> ()  [unwired: 2 in, 2 out]
                n140 = Wait (ms)(milliseconds to wait=w563) -> ()  [unwired: 1 out]
              }
              frame #3 {
                n141 = local write "Manual Script Entry (0)"(w569) -> ()
                n142 = local write "Script\n#"(w570) -> ()
              }
              frame #4 {
                n143 = local write "New Background Movie"(FALSE ("New Background Movie")) -> ()
              }
            }
            n144 = local read "Cycle time\n(ms)"() -> (w551:i32)
            n145 = local read "# Frames"() -> (w550:i32)
            n146 = local read "MODE"() -> (w549:u16)
            n147 = local read "BIN"() -> (w552:u16)
            n148 = call "BGScriptGenerator.vi"("Cycle time\n(ms)"=w551, "# Frames"=w550, "BIN"=w552, "MODE"=w549) -> ("Duration (ms)"=w542:i32, "BG Script"=w547:string)  [unwired: 6 in]
          }
        }
      }
    }
  }
  n149 = while {
    shift-right: [w670] -> w145
    shift-left: w144 -> [w669]
    shift-right: [w671] -> w146
    shift-left: w143 -> [w668]
    shift-right: [w665] -> w136
    shift-left: w141 -> [w667]
    shift-right: [w664] -> w135
    shift-left: w140 -> [w666]
    shift-right: [w663] -> w81
    shift-left: _ -> [w661]
    shift-right: [w662] -> w80
    shift-left: _ -> [w660]
    shift-right: [w657] -> w105
    shift-left: w116 -> [w659]
    shift-right: [w656] -> w107
    shift-left: w117 -> [w655]
    shift-right: [w653] -> w120
    shift-left: w130 -> [w654]
    shift-right: [w651] -> w121
    shift-left: w129 -> [w652]
    tunnel: w118 -> [w658]
    tunnel: [w627] -> w106
    shift-right: [w624] -> w85
    shift-left: w87 -> [w626]
    shift-right: [w623] -> w84
    shift-left: w86 -> [w625]
    shift-right: [w612] -> _
    shift-left: _ -> [w616]
    shift-right: [w611] -> w48
    shift-left: w46 -> [w608]
    shift-right: [w610] -> w49
    shift-left: w47 -> [w609]
    shift-right: [w602] -> w40
    shift-left: w44 -> [w605]
    shift-right: [w603] -> w39
    shift-left: w43 -> [w604]
    shift-right: [w596] -> _
    shift-left: _ -> [w598]
    shift-right: [w583] -> _
    shift-left: w24 -> [w585]
    shift-right: [w580] -> w15
    shift-left: w18 -> [w581]
    shift-right: [w579] -> w16
    shift-left: w19 -> [w582]
    stop <- w617 stop-if-true
    n150 = local read "DATA"() -> (w622:bool)
    n151 = Get Date/Time In Seconds() -> (seconds since 1Jan1904=w587:timestamp)
    n152 = call <instrlib>:"Collect Data.vi"("Location of FieldMax2Lib.dll in"=w625, "Meter ID in"=w626) -> ("Location of FieldMax2Lib.dll out"=w623:path, "Meter ID out"=w624:i32, "Measurement"=w620:sgl)  [unwired: 5 in, 1 out]
    n153 = Multiply(x="Data Interval (s)", y=u32 1000 ("millisecond multiple")) -> (x*y=w628:dbl)
    n154 = To Double Precision Float(number=w587) -> (double precision float=w583:dbl)
    n155 = Subtract(x=w583, y=w585) -> (x-y=w584:dbl)
    n156 = Multiply(x=w620, y=1000.0) -> (x*y=w619:dbl)
    "Power (mW)" <- w619
    n157 = Get Date/Time String(seconds (now)=w587, want seconds? (F)=TRUE) -> (time string=→"time string":string)  [unwired: 1 in, 1 out]
    n158 = call "Lakeshore218ReadTemp.vi"("error in"=w582, "VISA resource name"=w581) -> ("error out"=w579:errorcluster, "Thick Film R (Ohms)"=w578:string, "VISA resource name out"=w580:refnum<visa-resource-name>)  [unwired: 7 in]
    n159 = case shown="True" "RECORD" {
      tunnel: w661 -> [w723 _]
      tunnel: w660 -> [w724 _]
      tunnel: [w724 w729] -> w631
      tunnel: [w723 w728] -> w632
      frame False {
      }
      frame True {
        n160 = local read "SCRIPTING"() -> (w727:bool)
        n161 = local read "Script\n#"() -> (w726:i32)
        n162 = local write "RECORD"(FALSE ("RECORD")) -> ()
        n163 = call "DataHeader.vi"("Script #"=w726, "Scripting"=w727) -> ("error out"=w728:errorcluster, "Timestamp"=→"Timestamp":string, "refnum out"=w729:refnum<file>)  [unwired: 7 in]
      }
    }
    n164 = call "Lakeshore218Parse.vi"("Resistance String"=w578) -> ("Low Level (Ohms)"=w575:dbl, "High Level (Ohms)"=→"High Level\n(Ohms)":dbl)  [unwired: 9 in]
    "Low Level\n(Ohms)" <- w575
    n165 = call-poly <instrlib>:"Open.vi"("error in (no error)"=w668, "Device Identifier"="MB1.T1:TEMP", "Mercury Reference In"=w669) -> ("error out"=w644:errorcluster, "Mercury Reference Out"=w643:T4)  [unwired: 7 in]
    n166 = call-poly <instrlib>:"Signals (Read).vi"("error in"=w644, "Mercury Reference In"=w643) -> ("error out"=w641:errorcluster, "Temperature"=w595:dbl, "Mercury Reference Out"=w642:T4)  [unwired: 5 in, 2 out]
    "Cryostat (K)" <- w595
    n167 = call-poly <instrlib>:"Open.vi"("error in (no error)"=w641, "Device Identifier"="DB6.T1:TEMP", "Mercury Reference In"=w642) -> ("error out"=w639:errorcluster, "Mercury Reference Out"=w640:T4)  [unwired: 7 in]
    n168 = case shown="True" "AUTOFILL" {
      tunnel: w575 -> [_ w675]
      frame False {
      }
      frame True {
        n169 = Less?(x=w675, y="LL (Ohms)") -> (x < y?=w677:bool)
        n170 = case shown="True" w677 {
          selector: w677 -> [_ w678]
          frame False {
          }
          frame True {
            n171 = property on="REFILL" class="Bool (strict)"("Val(Sgnl)"=w678) -> ()  [unwired: 2 in, 2 out]
          }
        }
      }
    }
    n172 = call "PressureControl - 3He.vi"("error in (no error)"=w654, "VISA resource name"=w652) -> ("error out"=w653:errorcluster, "3HePressure (Torr)"=w589:string, "VISA resource name out"=w651:refnum<visa-resource-name>)  [unwired: 7 in]
    n173 = call "PressureControl - 4He.vi"("error in (no error)"=w667, "VISA resource name"=w666) -> ("error out"=w665:errorcluster, "Pressure"=w634:dbl, "Pressure (Torr)"=w590:string, "VISA resource name out"=w664:refnum<visa-resource-name>)  [unwired: 6 in]
    n174 = call-poly <instrlib>:"Signals (Read).vi"("error in"=w639, "Mercury Reference In"=w640) -> ("error out"=w671:errorcluster, "Temperature"=w633:dbl, "Mercury Reference Out"=w670:T4)  [unwired: 5 in, 2 out]
    "Cell (K)" <- w633
    n175 = case shown="\"Fill Tanks\"" "Turbulence" {
      tunnel: w590 -> [w731 w734]
      tunnel: w589 -> [w732 w733]
      frame "Main Controls", Default {
        "Tank Pressure 2 (Torr)" <- w732
        "Tank Pressure 1 (Torr)" <- w731
      }
      frame "Fill Tanks" {
        n176 = event shown="[2] \"3He Pressure (Torr)\": Value Change" {
          selector: _ -> [_ _ _ _]
          dyn-events: _ -> [_ _ _ _]
          timeout: 500 ("Numeric") -> [_ _ _ _]
          tunnel: w733 -> [_ _ _ w740]
          tunnel: w734 -> [_ _ _ w742]
          event Timeout {
            n177 = event-data() -> ()  [unwired: 1 in, 3 out]
          }
          event "Desired Tank\nPressure (3He)": Value Change {
            n178 = event-data() -> ("NewVal"=w736:dbl)  [unwired: 1 in]
            n179 = call "3HePressureCalculator.vi"("Desired Tank\nPressure (3He)"=w736) -> ("V2 Pressure (3He)"=→"Desired V2\nPressure (3He)":dbl)  [unwired: 10 in]
          }
          event "3He Pressure (Torr)": Value Change {
            n180 = event-data() -> ("NewVal"=w738:string)  [unwired: 1 in]
            n181 = call "3HeActualPressure.vi"("3He Pressure (Torr)"=w738) -> ("Actual 3He\nTank Pressure"=→"Actual 3He\nTank Pressure":dbl)  [unwired: 10 in]
          }
          event "Log Pressure": Value Change {
            n182 = event-data() -> ("NewVal"=w741:bool)  [unwired: 1 in]
            n183 = call "SaveTankData.vi"("Log Pressure"=w741, "4He Pressure (Torr)"=w742, "3He Pressure (Torr)"=w740) -> ()  [unwired: 8 in]
          }
        }
        "3He Pressure (Torr)" <- w733
        "4He Pressure (Torr)" <- w734
      }
    }
    n184 = call-poly <vilib>:"DAQmx Read.vi"("task/channels in"=w609, "error in"=w608) -> ("task out"=w607:refnum<k21>, "data"=w612:dbl, "error out"=w606:errorcluster)  [unwired: 11 in]
    "Detected" <- w612
    n185 = call-poly <vilib>:"DAQmx Read.vi"("task/channels in"=w605, "error in"=w604) -> ("task out"=w601:refnum<k21>, "data"=w596:dbl, "error out"=w600:errorcluster)  [unwired: 11 in]
    "Incident" <- w596
    n186 = case shown="True" w622 {
      tunnel: w655 -> [w682 w712]
      tunnel: w659 -> [w684 w711]
      tunnel: w658 -> [w683 w710]
      tunnel: [w683 w706] -> w638
      tunnel: [w682 w705] -> w637
      tunnel: [w684 w704] -> w636
      tunnel: w633 -> [_ w698]
      tunnel: w595 -> [_ w696]
      tunnel: w632 -> [w680 w695]
      tunnel: w590 -> [_ w694]
      tunnel: w631 -> [w681 w693]
      tunnel: [w680 w692] -> w630
      tunnel: [w681 w691] -> w629
      tunnel: w628 -> [w679 w689]
      tunnel: [w679 w688] -> w618
      tunnel: w619 -> [_ w687]
      tunnel: w612 -> [_ w686]
      tunnel: w596 -> [_ w685]
      frame False {
      }
      frame True {
        n187 = Subtract(x=w689, y=350.0) -> (x-y=w688:dbl)
        n188 = call <instrlib>:"Measure.vi"("Function (Current)"=T6."Power", "error in (no error)"=w712, "Node In"=w710, "VISA resource name"=w711) -> ("error out"=w703:errorcluster, "Output"=w697:string, "Node Out"=w707:string, "VISA resource name out"=w708:refnum<visa-resource-name>)  [unwired: 3 in, 1 out]
        n189 = flat-sequence {
          tunnel: w703 -> [w713]
          tunnel: [w713] -> w702
          frame #0 {
            n190 = Wait (ms)(milliseconds to wait=u32 100) -> ()  [unwired: 1 out]
          }
        }
        n191 = call <instrlib>:"Measure.vi"("Function (Current)"=T6."Power", "error in (no error)"=w702, "Channel (Channel A)"=Channel."Channel B", "Node In"=w707, "VISA resource name"=w708) -> ("error out"=w705:errorcluster, "Output"=w699:string, "Node Out"=w706:string, "VISA resource name out"=w704:refnum<visa-resource-name>)  [unwired: 2 in, 1 out]
        n192 = call "CompileData.vi"("Detected"=w686, "Incident"=w685, "Ch. B (W)"=w699, "Cell Temp (K)"=w698, "Ch. A (W)"=w697, "Cryostat Temp (K)"=w696, "error in"=w695, "Laser Power (W)"=w687, "Tank Pressure (Torr)"=w694, "refnum in"=w693) -> ("error out"=w692:errorcluster, "refnum out"=w691:refnum<file>)
      }
    }
    n193 = case shown="True" "CLOSE" {
      tunnel: w630 -> [w715 w721]
      tunnel: w629 -> [w716 w720]
      tunnel: [w716 refnum<file> refnum ("refnum out")] -> w662
      tunnel: [w715 errorcluster {"status"=FALSE, "code"=0, "source"=""} ("error out")] -> w663
      frame False {
      }
      frame True {
        n194 = local write "CLOSE"(FALSE ("CLOSE")) -> ()
        n195 = Close File(refnum=w720, error in=w721) -> (error out=→"File I/O Error":errorcluster)  [unwired: 1 out]
      }
    }
    n196 = Less?(x=w595, y=2.17) -> (x < y?=w592:bool)
    n197 = event shown="[5] \"RESTART\": Value Change" {
      selector: _ -> [_ _ _ _ _ _]
      dyn-events: _ -> [_ _ _ _ _ _]
      timeout: w618 -> [_ _ _ _ _ _]
      tunnel: w638 -> [w747 w761 w773 w785 w797 w810]
      tunnel: w637 -> [w748 w762 w775 w787 w799 w811]
      tunnel: w636 -> [w749 w760 w772 w784 w796 w809]
      tunnel: [w749 w759 w774 w786 w798 w809] -> w657
      tunnel: [w748 w755 w768 w782 w793 w811] -> w656
      tunnel: [w747 w754 w767 w781 w792 w810] -> w627
      tunnel: [w746 w753 w766 w780 w791 w808] -> w611
      tunnel: [w745 w752 w765 w779 w790 w807] -> w610
      tunnel: w607 -> [w745 w752 w765 w779 w790 w806]
      tunnel: w606 -> [w746 w753 w766 w780 w791 w805]
      tunnel: [w744 w751 w764 w778 w789 w803] -> w602
      tunnel: [w743 w750 w763 w777 w788 w802] -> w603
      tunnel: w601 -> [w744 w751 w764 w778 w789 w801]
      tunnel: w600 -> [w743 w750 w763 w777 w788 w800]
      event Timeout {
        n198 = event-data() -> ()  [unwired: 1 in, 3 out]
      }
      event "Top Coil (mA)": Value Change {
        n199 = event-data() -> ("NewVal"=w757:dbl)  [unwired: 1 in, 5 out]
        n200 = Divide(x=w757, y=1000.0) -> (x/y=w756:dbl)
        n201 = call <instrlib>:"Source Level.vi"("Level (0.000)"=w756, "error in (no error)"=w762, "Node In"=w761, "VISA resource name"=w760) -> ("error out"=w755:errorcluster, "Node Out"=w754:string, "VISA resource name out"=w759:refnum<visa-resource-name>)  [unwired: 4 in, 1 out]
      }
      event "Bottom Coil (mA)": Value Change {
        n202 = event-data() -> ("NewVal"=w770:dbl)  [unwired: 1 in, 5 out]
        n203 = Divide(x=w770, y=1000.0) -> (x/y=w769:dbl)
        n204 = call <instrlib>:"Source Level.vi"("Level (0.000)"=w769, "error in (no error)"=w775, "Channel (Channel A)"=Channel."Channel B", "Node In"=w773, "VISA resource name"=w772) -> ("error out"=w768:errorcluster, "Node Out"=w767:string, "VISA resource name out"=w774:refnum<visa-resource-name>)  [unwired: 3 in, 1 out]
      }
      event "Top Coil": Value Change {
        n205 = event-data() -> ("NewVal"=w783:bool)  [unwired: 1 in, 5 out]
        n206 = call <instrlib>:"Source Output Enable.vi"("Output (Off)"=w783, "error in (no error)"=w787, "Node In"=w785, "VISA resource name"=w784) -> ("error out"=w782:errorcluster, "Node Out"=w781:string, "VISA resource name out"=w786:refnum<visa-resource-name>)  [unwired: 4 in, 1 out]
      }
      event "Bottom Coil": Value Change {
        n207 = event-data() -> ("NewVal"=w794:bool)  [unwired: 1 in, 5 out]
        n208 = call <instrlib>:"Source Output Enable.vi"("Output (Off)"=w794, "error in (no error)"=w799, "Channel (Channel A)"=Channel."Channel B", "Node In"=w797, "VISA resource name"=w796) -> ("error out"=w793:errorcluster, "Node Out"=w792:string, "VISA resource name out"=w798:refnum<visa-resource-name>)  [unwired: 3 in, 1 out]
      }
      event "RESTART": Value Change {
        n209 = event-data() -> ("NewVal"=w804:bool)  [unwired: 1 in, 5 out]
        n210 = case shown="True" w804 {
          tunnel: w806 -> [w815 w825]
          tunnel: w805 -> [w814 w826]
          tunnel: [w815 w824] -> w807
          tunnel: [w814 w823] -> w808
          tunnel: [w813 w819] -> w803
          tunnel: [w812 w818] -> w802
          tunnel: w801 -> [w813 w817]
          tunnel: w800 -> [w812 w816]
          frame False {
          }
          frame True {
            n211 = call <vilib>:"DAQmx Stop Task.vi"("task/channels in"=w825, "error in"=w826) -> ("task out"=w822:refnum<k21>, "error out"=w827:errorcluster)  [unwired: 12 in]
            n212 = call <vilib>:"DAQmx Stop Task.vi"("task/channels in"=w817, "error in"=w816) -> ("task out"=w820:refnum<k21>, "error out"=w821:errorcluster)  [unwired: 12 in]
            n213 = local write "RESTART"(FALSE ("RESTART")) -> ()
            n214 = call <vilib>:"DAQmx Start Task.vi"("task/channels in"=w822, "error in"=w827) -> ("task out"=w824:refnum<k21>, "error out"=w823:errorcluster)  [unwired: 12 in]
            n215 = call <vilib>:"DAQmx Start Task.vi"("task/channels in"=w820, "error in"=w821) -> ("task out"=w819:refnum<k21>, "error out"=w818:errorcluster)  [unwired: 12 in]
          }
        }
      }
    }
    n216 = Subtract(x=w596, y=w598) -> (x-y=w597:dbl)
    n217 = Subtract(x=w612, y=w616) -> (x-y=w615:dbl)
    n218 = Less?(x=w634, y=24.5) -> (x < y?=w593:bool)
    n219 = And(x=w592, y=w593) -> (x .and. y?=w591:bool)
    n220 = Divide(x=w597, y=w584) -> (x/y=→"Rate (Hz)":dbl)
    n221 = Divide(x=w615, y=w584) -> (x/y=→"Rate (Hz)":dbl)
    n222 = case shown="True" w591 {
      tunnel: [FALSE ("RUN/STOP") TRUE ("RUN/STOP")] -> w572
      frame False {
      }
      frame True {
      }
    }
    n223 = property on="READY" class="Bool (strict)"() -> ("Value"=w574:bool)  [unwired: 2 in, 2 out]
    n224 = Equal?(x=w574, y=w572) -> (x = y?=w573:bool)
    n225 = case shown="False" w573 {
      tunnel: w572 -> [w672 _]
      frame False {
        n226 = property on="READY" class="Bool (strict)"("Val(Sgnl)"=w672) -> ()  [unwired: 2 in, 2 out]
      }
      frame True {
      }
    }
    n227 = local read "Kill Switch"() -> (w617:bool)
  }
  n228 = local write "3He Check"(TRUE ("3He Check")) -> ()
  n229 = call "LogHeader.vi"("Data folder"=path "C:/Data") -> ("error out"=w76:errorcluster, "refnum out"=w77:refnum<file>)  [unwired: 9 in]
  "Log" <- w77
  n230 = call "MFCInit.vi"() -> ("MFC error out"=w11:errorcluster, "MFC VISA out"=w10:refnum<visa-resource-name>)  [unwired: 10 in]
  n231 = local write "Error"(FALSE ("Error")) -> ()
  n232 = while {
    tunnel: [w829] -> w3
    stop <- w831 stop-if-true
    n233 = event shown="[1] \"FROM FILE\": Value Change" {
      selector: _ -> [_ _]
      dyn-events: _ -> [_ _]
      timeout: 500 -> [_ _]
      tunnel: [i32[] [] w833] -> w829
      event Timeout {
        n234 = event-data() -> ()  [unwired: 1 in, 3 out]
      }
      event "FROM FILE": Value Change {
        n235 = event-data() -> ("NewVal"=w834:bool)  [unwired: 1 in]
        n236 = case shown="True" w834 {
          tunnel: [i32[] [] w836] -> w833
          frame False {
          }
          frame True {
            n237 = call "ScriptReader.vi"("Script File"="Script File") -> ("Different Scripts"=w838:i32, "Scripts"=w839:i32[][])  [unwired: 9 in]
            n238 = for {
              N: w838 -> [_]
              tunnel: w839 -> [w847] mode=indexing
              tunnel: [w843] -> w837 mode=indexing
              stop <- w852 stop-if-true
              n239 = Index Array(array=w847, index=0) -> (element=w848:i32)
              n240 = Index Array(array=w847, index=1) -> (element=w846:i32)
              n241 = local write "Script\nEnd"(w848) -> ()
              n242 = local write "Script\n#"(w848) -> ()
              n243 = while {
                shift-right: [w856] -> w843
                shift-left: w846 -> [w854]
                stop <- w861 stop-if-true
                n244 = flat-sequence {
                  tunnel: w854 -> [w864]
                  tunnel: [w864] -> w857
                  tunnel: w857 -> [w870]
                  tunnel: [w867] -> w856
                  frame #0 {
                    n245 = property on="SCRIPTING" class="Bool (strict)"("Val(Sgnl)"=TRUE ("Value (Signaling)")) -> ()  [unwired: 2 in, 2 out]
                    n246 = local write "Error"(FALSE ("Error")) -> ()
                  }
                  frame #1 {
                    n247 = while {
                      tunnel: [w909] -> w869
                      tunnel: w870 -> [w909]
                      tunnel: [w908] -> w868
                      tunnel: [w903] -> w866
                      stop <- w905 stop-if-true
                      n248 = local read "FROM FILE"() -> (w911:bool)
                      n249 = local read "SCRIPTING"() -> (w904:bool)
                      n250 = local read "Kill Switch"() -> (w910:bool)
                      n251 = local read "READY"() -> (w913:bool)
                      n252 = Not(x=w911) -> (.not. x?=w912:bool)
                      n253 = Not(x=w904) -> (.not. x?=w903:bool)
                      n254 = Not(x=w913) -> (.not. x?=w908:bool)
                      n255 = Or(x=w908, y=w912) -> (x .or. y?=w914:bool)
                      n256 = Or(x=w914, y=w910) -> (x .or. y?=w906:bool)
                      n257 = Or(x=w903, y=w906) -> (x .or. y?=w905:bool)
                      n258 = Wait (ms)(milliseconds to wait=u32 1000) -> ()  [unwired: 1 out]
                    }
                    n259 = case shown="True" w868 {
                      tunnel: w869 -> [w873 w881]
                      tunnel: [w872 w881] -> w867
                      tunnel: w866 -> [w871 _]
                      frame False {
                        n260 = case shown="True" w871 {
                          tunnel: w873 -> [w874 w877]
                          tunnel: [w874 w876] -> w872
                          frame False {
                          }
                          frame True {
                            n261 = Decrement(x=w877) -> (x-1=w876:i32)
                            n262 = Wait (ms)(milliseconds to wait=u32 13000) -> ()  [unwired: 1 out]
                          }
                        }
                      }
                      frame True {
                        n263 = local write "Error"(TRUE ("Error")) -> ()
                        n264 = while {
                          tunnel: [w893] -> w880
                          tunnel: [w892] -> w878
                          i -> [w899]
                          stop <- w900 stop-if-true
                          n265 = local read "Kill Switch"() -> (w894:bool)
                          n266 = local read "FROM FILE"() -> (w896:bool)
                          n267 = local read "READY"() -> (w892:bool)
                          n268 = Equal?(x=w899, y=60) -> (x = y?=w893:bool)
                          n269 = Not(x=w896) -> (.not. x?=w895:bool)
                          n270 = Or(x=w894, y=w893) -> (x .or. y?=w897:bool)
                          n271 = Or(x=w895, y=w897) -> (x .or. y?=w901:bool)
                          n272 = Or(x=w901, y=w892) -> (x .or. y?=w900:bool)
                          n273 = Wait (ms)(milliseconds to wait=u32 1000) -> ()  [unwired: 1 out]
                        }
                        n274 = case shown="False" w880 {
                          selector: w880 -> [_ w884]
                          tunnel: w878 -> [w882 _]
                          frame False {
                            n275 = case shown="True" w882 {
                              frame False {
                              }
                              frame True {
                                n276 = Wait (ms)(milliseconds to wait=u32 13000) -> ()  [unwired: 1 out]
                              }
                            }
                          }
                          frame True {
                            n277 = property on="COOLDOWN" class="Bool (strict)"("Val(Sgnl)"=w884) -> ()  [unwired: 2 in, 2 out]
                            n278 = while {
                              stop <- w890 stop-if-true
                              n279 = local read "Kill Switch"() -> (w888:bool)
                              n280 = local read "READY"() -> (w885:bool)
                              n281 = local read "FROM FILE"() -> (w886:bool)
                              n282 = Not(x=w886) -> (.not. x?=w887:bool)
                              n283 = Or(x=w885, y=w888) -> (x .or. y?=w889:bool)
                              n284 = Or(x=w889, y=w887) -> (x .or. y?=w890:bool)
                              n285 = Wait (ms)(milliseconds to wait=u32 1000) -> ()  [unwired: 1 out]
                            }
                          }
                        }
                      }
                    }
                  }
                }
                n286 = local read "Kill Switch"() -> (w862:bool)
                n287 = local read "FROM FILE"() -> (w859:bool)
                n288 = Equal?(x=1, y=w854) -> (x = y?=w855:bool)
                n289 = Or(x=w862, y=w855) -> (x .or. y?=w860:bool)
                n290 = Not(x=w859) -> (.not. x?=w858:bool)
                n291 = Or(x=w860, y=w858) -> (x .or. y?=w861:bool)
              }
              n292 = local read "FROM FILE"() -> (w844:bool)
              n293 = local read "Kill Switch"() -> (w851:bool)
              n294 = Not(x=w844) -> (.not. x?=w845:bool)
              n295 = Or(x=w845, y=w851) -> (x .or. y?=w852:bool)
            }
            n296 = flat-sequence {
              tunnel: w837 -> [w841]
              tunnel: [w841] -> w836
              frame #0 {
                n297 = property on="FROM FILE" class="Bool (strict)"("Val(Sgnl)"=FALSE ("Value (Signaling)")) -> ()  [unwired: 2 in, 2 out]
              }
            }
          }
        }
      }
    }
    n298 = local read "Kill Switch"() -> (w831:bool)
  }
  n299 = while {
    shift-right: [w925] -> w75
    shift-left: w77 -> [w926]
    shift-right: [w924] -> w74
    shift-left: w76 -> [w927]
    shift-right: [w918] -> w7
    shift-left: w10 -> [w922]
    shift-right: [w919] -> w8
    shift-left: w11 -> [w923]
    shift-right: [w920] -> _
    shift-left: 0.0 ("3He Pressure") -> [w921]
    stop <- w917 stop-if-true
    n300 = event shown="[0] \"SCRIPTING\": Value Change" {
      selector: _ -> [_ _ _ _]
      dyn-events: _ -> [_ _ _ _]
      timeout: 500 -> [_ _ _ _]
      tunnel: w927 -> [w935 w1425 w1498 w1512]
      tunnel: w926 -> [w936 w1424 w1499 w1513]
      tunnel: [w934 w1424 w1499 w1513] -> w925
      tunnel: [w933 w1425 w1498 w1512] -> w924
      tunnel: w923 -> [w930 w1430 w1502 w1510]
      tunnel: w922 -> [w929 w1431 w1503 w1509]
      tunnel: w921 -> [w931 w1429 w1501 w1511]
      tunnel: [w931 w1428 w1500 w1511] -> w920
      tunnel: [w930 w1427 w1502 w1510] -> w919
      tunnel: [w929 w1426 w1503 w1509] -> w918
      event "SCRIPTING": Value Change {
        n301 = event-data() -> ()  [unwired: 1 in, 1 out]
        n302 = case shown="True" "SCRIPTING" {
          tunnel: w936 -> [w938 w942]
          tunnel: w935 -> [w937 w941]
          tunnel: [w938 w939] -> w934
          tunnel: [w937 w940] -> w933
          frame False {
          }
          frame True {
            n303 = local read "Script\n#"() -> (w944:i32)
            n304 = Not Equal To 0?(x=w944) -> (x != 0?=w943:bool)
            n305 = case shown="True" w943 {
              tunnel: w942 -> [w950 w1134]
              tunnel: w941 -> [w951 w1135]
              tunnel: [w945 w1132] -> w940
              tunnel: [w946 w1133] -> w939
              frame False {
                n306 = call "GetManualCommands.vi"("Manual Script Entry (0)"="Manual Script Entry (0)") -> ("Commands"=w958:string[])  [unwired: 10 in]
                n307 = Array Size(array=w958) -> (size(s)=w954:i32)
                n308 = for {
                  tunnel: w958 -> [w990] mode=indexing
                  tunnel: [w985] -> w957
                  tunnel: [w984] -> w952
                  i -> [w985]
                  stop <- w987 stop-if-true
                  n309 = Match Pattern(string=w990, regular expression="[a-z]+") -> (match substring=w983:string, after substring=w982:string)  [unwired: 1 in, 2 out]
                  n310 = call <vilib>:"Trim Whitespace.vi"("string"=w982) -> ("trimmed string"=w989:string)  [unwired: 1 in]
                  n311 = Concatenate Strings(w983, w982) -> (w981:string)
                  n312 = case shown="\"data\"" w983 {
                    tunnel: w989 -> [_ w1003 w1022 w1037 w1044 w1062 w1080 w1109]
                    tunnel: [TRUE ("Top Coil") w1002 w1019 FALSE ("Top Coil") w1041 w1059 w1079 w1108] -> w986
                    tunnel: w985 -> [w995 w1001 w1021 _ w1043 w1061 w1078 w1107]
                    tunnel: u32 0 ("Script Number") -> [w994 w1000 w1020 _ w1042 w1060 w1077 w1106]
                    tunnel: [w993 w998 w1017 "" ("Error String") w1039 w1058 w1075 w1104] -> w984
                    tunnel: w981 -> [w992 w997 w1016 _ w1038 w1057 w1074 w1103]
                    frame "False", Default {
                      n313 = call "ErrorHandling.vi"("Bad Command"=w992, "Line #"=w995, "Script #"=w994) -> ("Error String"=w993:string)  [unwired: 8 in]
                    }
                    frame "data" {
                      n314 = case shown="\"False\", Default" w1003 {
                        tunnel: [FALSE ("DATA") TRUE ("DATA") FALSE ("DATA")] -> w999
                        tunnel: [TRUE ("Top Coil") FALSE ("Top Coil") FALSE ("Top Coil")] -> w1002
                        tunnel: w1001 -> [w1006 _ _]
                        tunnel: w1000 -> [w1007 _ _]
                        tunnel: [w1005 "" ("Error String") "" ("Error String")] -> w998
                        tunnel: w997 -> [w1004 _ _]
                        frame "False", Default {
                          n315 = call "ErrorHandling.vi"("Bad Command"=w1004, "Line #"=w1006, "Script #"=w1007) -> ("Error String"=w1005:string)  [unwired: 8 in]
                        }
                        frame "on" {
                        }
                        frame "off" {
                        }
                      }
                      n316 = property on="DATA" class="Bool (strict)"("Val(Sgnl)"=w999) -> ()  [unwired: 2 in, 2 out]
                    }
                    frame "pulse" {
                      n317 = case shown="\"False\", Default" w1022 {
                        tunnel: [FALSE ("Top Coil") TRUE ("Top Coil") w1033] -> w1018
                        tunnel: [TRUE FALSE w1033] -> w1019
                        tunnel: w1021 -> [w1026 _ _]
                        tunnel: w1020 -> [w1025 _ _]
                        tunnel: [w1024 "" ""] -> w1017
                        tunnel: w1016 -> [w1023 _ _]
                        frame "False", Default {
                          n318 = call "ErrorHandling.vi"("Bad Command"=w1023, "Line #"=w1026, "Script #"=w1025) -> ("Error String"=w1024:string)  [unwired: 8 in]
                        }
                        frame "on" {
                        }
                        frame "off" {
                          w1033 = FALSE ("Top Coil")
                        }
                      }
                      n319 = property on="RUN/STOP" class="Bool (strict)"("Val(Sgnl)"=w1018) -> ()  [unwired: 2 in, 2 out]
                    }
                    frame "wait" {
                      n320 = Decimal String To Number(string=w1037) -> (number=w1036:i32)  [unwired: 2 in, 1 out]
                      n321 = Wait (ms)(milliseconds to wait=w1036) -> ()  [unwired: 1 out]
                    }
                    frame "neutron" {
                      n322 = case shown="\"False\", Default" w1044 {
                        tunnel: w1043 -> [w1050 _ _]
                        tunnel: w1042 -> [w1049 _ _]
                        tunnel: [TRUE ("Top Coil") FALSE ("Top Coil") w1055] -> w1041
                        tunnel: [FALSE ("Neutron Shutter") TRUE ("Neutron Shutter") w1055] -> w1040
                        tunnel: [w1046 "" ("Error String") "" ("Error String")] -> w1039
                        tunnel: w1038 -> [w1045 _ _]
                        frame "False", Default {
                          n323 = call "ErrorHandling.vi"("Bad Command"=w1045, "Line #"=w1050, "Script #"=w1049) -> ("Error String"=w1046:string)  [unwired: 8 in]
                        }
                        frame "on" {
                        }
                        frame "off" {
                          w1055 = FALSE ("Neutron Shutter")
                        }
                      }
                      n324 = property on="Neutron Shutter" class="Bool (strict)"("Val(Sgnl)"=w1040) -> ()  [unwired: 2 in, 2 out]
                    }
                    frame "shutter" {
                      n325 = case shown="\"False\", Default" w1062 {
                        tunnel: w1061 -> [w1068 _ _]
                        tunnel: w1060 -> [w1067 _ _]
                        tunnel: [TRUE ("Top Coil") FALSE ("Top Coil") w1073] -> w1059
                        tunnel: [FALSE ("Neutron Shutter") TRUE ("Neutron Shutter") w1073] -> w1056
                        tunnel: [w1064 "" ("Error String") "" ("Error String")] -> w1058
                        tunnel: w1057 -> [w1063 _ _]
                        frame "False", Default {
                          n326 = call "ErrorHandling.vi"("Bad Command"=w1063, "Line #"=w1068, "Script #"=w1067) -> ("Error String"=w1064:string)  [unwired: 8 in]
                        }
                        frame "on" {
                        }
                        frame "off" {
                          w1073 = FALSE ("Neutron Shutter")
                        }
                      }
                      n327 = property on="Enable" class="Bool (strict)"("Val(Sgnl)"=w1056) -> ()  [unwired: 2 in, 2 out]
                    }
                    frame "coila" {
                      n328 = case shown="\"False\", Default" w1080 {
                        selector: w1080 -> [w1087 _]
                        tunnel: [w1089 w1102] -> w1076
                        tunnel: [w1088 w1102] -> w1079
                        tunnel: w1078 -> [w1084 _]
                        tunnel: w1077 -> [w1083 _]
                        tunnel: [w1082 "" ("Error String")] -> w1075
                        tunnel: w1074 -> [w1081 _]
                        frame "False", Default {
                          n329 = Match Pattern(string=w1087, regular expression="[^0-9.]") -> (offset past match=w1085:i32)  [unwired: 1 in, 3 out]
                          n330 = case shown="0, Default" w1085 {
                            tunnel: [FALSE ("Top Coil") TRUE ("Top Coil")] -> w1089
                            tunnel: [TRUE FALSE] -> w1088
                            tunnel: w1087 -> [_ w1098]
                            tunnel: w1084 -> [w1093 _]
                            tunnel: w1083 -> [w1092 _]
                            tunnel: [w1091 ""] -> w1082
                            tunnel: w1081 -> [w1090 _]
                            frame 0, Default {
                              n331 = call "ErrorHandling.vi"("Bad Command"=w1090, "Line #"=w1093, "Script #"=w1092) -> ("Error String"=w1091:string)  [unwired: 8 in]
                            }
                            frame -1 {
                              n332 = Fract/Exp String To Number(string=w1098) -> (number=w1097:dbl)  [unwired: 3 in, 1 out]
                              n333 = property on="Top Coil (mA)" class="DigNum (strict)"("Val(Sgnl)"=w1097) -> ()  [unwired: 2 in, 2 out]
                            }
                          }
                        }
                        frame "off" {
                          w1102 = FALSE ("Top Coil")
                        }
                      }
                      n334 = property on="Top Coil" class="Bool (strict)"("Val(Sgnl)"=w1076) -> ()  [unwired: 2 in, 2 out]
                    }
                    frame "coilb" {
                      n335 = case shown="\"False\", Default" w1109 {
                        selector: w1109 -> [w1116 _]
                        tunnel: [w1115 w1131] -> w1105
                        tunnel: [w1114 w1131] -> w1108
                        tunnel: w1107 -> [w1113 _]
                        tunnel: w1106 -> [w1112 _]
                        tunnel: [w1111 ""] -> w1104
                        tunnel: w1103 -> [w1110 _]
                        frame "False", Default {
                          n336 = Match Pattern(string=w1116, regular expression="[^0-9.]") -> (offset past match=w1117:i32)  [unwired: 1 in, 3 out]
                          n337 = case shown="0, Default" w1117 {
                            tunnel: w1116 -> [_ w1129]
                            tunnel: [FALSE TRUE] -> w1115
                            tunnel: [TRUE FALSE] -> w1114
                            tunnel: w1113 -> [w1122 _]
                            tunnel: w1112 -> [w1121 _]
                            tunnel: [w1120 ""] -> w1111
                            tunnel: w1110 -> [w1119 _]
                            frame 0, Default {
                              n338 = call "ErrorHandling.vi"("Bad Command"=w1119, "Line #"=w1122, "Script #"=w1121) -> ("Error String"=w1120:string)  [unwired: 8 in]
                            }
                            frame -1 {
                              n339 = Fract/Exp String To Number(string=w1129) -> (number=w1126:dbl)  [unwired: 3 in, 1 out]
                              n340 = property on="Bottom Coil (mA)" class="DigNum (strict)"("Val(Sgnl)"=w1126) -> ()  [unwired: 2 in, 2 out]
                            }
                          }
                        }
                        frame "off" {
                          w1131 = FALSE
                        }
                      }
                      n341 = property on="Bottom Coil" class="Bool (strict)"("Val(Sgnl)"=w1105) -> ()  [unwired: 2 in, 2 out]
                    }
                  }
                  n342 = local read "Kill Switch"() -> (w980:bool)
                  n343 = Or(x=w986, y=w980) -> (x .or. y?=w987:bool)
                }
                n344 = Decrement(x=w954) -> (x-1=w956:i32)
                n345 = Equal?(x=w957, y=w956) -> (x = y?=w955:bool)
                n346 = case shown="False" w955 {
                  tunnel: [w974 w977] -> w953
                  tunnel: w952 -> [w972 _]
                  tunnel: [w970 w976] -> w948
                  frame False {
                    w969 = FALSE ("status")
                    n347 = property on="Bottom Coil" class="Bool (strict)"("Val(Sgnl)"=w969) -> ()  [unwired: 2 in, 2 out]
                    n348 = property on="Neutron Shutter" class="Bool (strict)"("Val(Sgnl)"=w969) -> ()  [unwired: 2 in, 2 out]
                    n349 = property on="Top Coil" class="Bool (strict)"("Val(Sgnl)"=w969) -> ()  [unwired: 2 in, 2 out]
                    n350 = property on="Enable" class="Bool (strict)"("Val(Sgnl)"=w969) -> ()  [unwired: 2 in, 2 out]
                    n351 = property on="RUN/STOP" class="Bool (strict)"("Val(Sgnl)"=w969) -> ()  [unwired: 2 in, 2 out]
                    n352 = property on="DATA" class="Bool (strict)"("Val(Sgnl)"=w969) -> ()  [unwired: 2 in, 2 out]
                    n353 = Concatenate Strings("Manual test failed!" ("Description"), "\r\n", w972) -> (w970:string)
                    n354 = Bundle("status"=w969, "code"=1017, w970) -> (w974:cluster{"status":bool, "code":i32, string})  [unwired: 1 in]
                  }
                  frame True {
                    w976 = "Manual test successful!" ("Description")
                    n355 = Bundle("status"=FALSE, "code"=0, "Description"=w976) -> (w977:T2)  [unwired: 1 in]
                  }
                }
                n356 = flat-sequence {
                  tunnel: w953 -> [w966]
                  tunnel: w951 -> [w962]
                  tunnel: w950 -> [w965]
                  tunnel: "Manual Script Entry (0)" -> [w964]
                  tunnel: w948 -> [w963]
                  tunnel: [w961] -> w947
                  tunnel: [w960] -> w945
                  tunnel: w947 -> [w968]
                  tunnel: [w968] -> w946
                  frame #0 {
                    n357 = local write "Scripting Error"(w966) -> ()
                    n358 = local read "Timestamp"() -> (w959:string)
                    n359 = call "WriteResults_Manual.vi"("Timestamp"=w959, "error in"=w962, "Result"=w963, "Commands"=w964, "refnum in"=w965) -> ("error out"=w960:errorcluster, "refnum out"=w961:refnum<file>)  [unwired: 5 in]
                  }
                  frame #1 {
                    n360 = property on="SCRIPTING" class="Bool (strict)"("Val(Sgnl)"=FALSE ("Value (Signaling)")) -> ()  [unwired: 2 in, 2 out]
                  }
                }
              }
              frame True {
                n361 = while {
                  tunnel: w1135 -> [w1141]
                  tunnel: w1134 -> [w1140]
                  tunnel: [w1139] -> w1133
                  tunnel: [w1137] -> w1132
                  stop <- w1136 stop-if-true
                  n362 = local read "Script\n#"() -> (w1143:i32)
                  n363 = call "GetCommands.vi"("Script Number"=w1143) -> ("Script Exists"=w1144:bool, "Commands"=w1145:string[], "Camera Settings"=w1146:dbl[], "Data Interval (s)"=w1142:dbl)  [unwired: 5 in]
                  n364 = case shown="True" w1144 {
                    tunnel: w1146 -> [_ w1184]
                    tunnel: w1145 -> [_ w1182]
                    tunnel: w1143 -> [w1163 w1180]
                    tunnel: w1142 -> [_ w1179]
                    tunnel: w1141 -> [w1157 w1177]
                    tunnel: w1140 -> [w1158 w1176]
                    tunnel: [w1156 w1175] -> w1139
                    tunnel: [w1155 w1174] -> w1138
                    frame False {
                      n365 = Number To Decimal String(number=w1163) -> (decimal integer string=w1162:string)  [unwired: 1 in]
                      n366 = Concatenate Strings("Script" ("string"), w1162, " does not exist." ("string")) -> (w1159:string)
                      n367 = Bundle("status"=FALSE, "code"=1017, w1159) -> (w1164:cluster{"status":bool, "code":i32, string})  [unwired: 1 in]
                      n368 = Get Date/Time In Seconds() -> (seconds since 1Jan1904=w1154:timestamp)
                      n369 = Format Date/Time String(time format string (%c)="%H:%M:%S", seconds (now)=w1154) -> (date/time string=w1152:string)  [unwired: 1 in]
                      n370 = local write "Scripting Error"(w1164) -> ()
                      n371 = call "WriteResults_Script.vi"("Timestamp"=w1152, "error in"=w1157, "Result"=w1159, "refnum in"=w1158) -> ("error out"=w1155:errorcluster, "refnum out"=w1156:refnum<file>)  [unwired: 6 in]
                      n372 = property on="SCRIPTING" class="Bool (strict)"("Val(Sgnl)"=FALSE ("Value (Signaling)")) -> ()  [unwired: 2 in, 2 out]
                    }
                    frame True {
                      n373 = flat-sequence {
                        tunnel: u32 100 ("milliseconds to wait") -> [w1193]
                        tunnel: w1184 -> [w1194]
                        tunnel: [w1194] -> w1173
                        tunnel: [w1193] -> w1172
                        tunnel: w1179 -> [w1192]
                        tunnel: w1173 -> [w1198]
                        tunnel: [w1198] -> w1191
                        tunnel: w1172 -> [w1197]
                        tunnel: [w1197] -> w1190
                        tunnel: w1191 -> [w1203]
                        tunnel: [w1203] -> w1189
                        tunnel: w1190 -> [w1202]
                        tunnel: [w1202] -> w1188
                        tunnel: w1189 -> [w1207]
                        tunnel: [w1207] -> w1171
                        tunnel: w1188 -> [w1206]
                        tunnel: [w1206] -> w1170
                        tunnel: w1171 -> [w1211]
                        tunnel: w1170 -> [w1212]
                        tunnel: [w1212] -> w1169
                        tunnel: [w1211] -> w1168
                        tunnel: [w1215] -> w1187
                        tunnel: w1169 -> [w1214]
                        tunnel: [w1214] -> w1186
                        tunnel: w1168 -> [w1215]
                        tunnel: w1187 -> [w1220]
                        tunnel: w1186 -> [w1219]
                        tunnel: w1182 -> [w1225]
                        tunnel: w1180 -> [w1224]
                        tunnel: [w1223] -> w1185
                        tunnel: [w1222] -> w1178
                        tunnel: w1181 -> [w1392]
                        tunnel: w1185 -> [w1393]
                        tunnel: w1180 -> [w1382]
                        tunnel: w1178 -> [w1389]
                        tunnel: w1177 -> [w1386]
                        tunnel: w1176 -> [w1387]
                        tunnel: [w1385] -> w1175
                        tunnel: [w1384] -> w1174
                        frame #0 {
                          n374 = property on="Data Interval (s)" class="DigNum (strict)"("Val(Sgnl)"=w1192) -> ()  [unwired: 2 in, 2 out]
                        }
                        frame #1 {
                          n375 = Index Array(array=w1198, index=0) -> (element=w1196:dbl)
                          n376 = To Unsigned Word Integer(number=w1196) -> (unsigned 16bit integer=w1195:u16)
                          n377 = local write "MODE"(w1195) -> ()
                        }
                        frame #2 {
                          n378 = Index Array(array=w1203, index=1) -> (element=w1201:dbl)
                          n379 = To Unsigned Word Integer(number=w1201) -> (unsigned 16bit integer=w1200:u16)
                          n380 = local write "BIN"(w1200) -> ()
                        }
                        frame #3 {
                          n381 = Index Array(array=w1207, index=2) -> (element=w1205:dbl)
                          n382 = local write "On CCD Acc."(w1205) -> ()
                        }
                        frame #4 {
                          n383 = Index Array(array=w1211, index=3) -> (element=w1209:dbl)
                          n384 = local write "Cycle time\n(ms)"(w1209) -> ()
                        }
                        frame #5 {
                          n385 = Index Array(array=w1215, index=4) -> (element=w1213:dbl)
                          n386 = property on="# Frames" class="DigNum (strict)"("Val(Sgnl)"=w1213) -> ()  [unwired: 2 in, 2 out]
                          n387 = Wait (ms)(milliseconds to wait=w1214) -> ()  [unwired: 1 out]
                        }
                        frame #6 {
                          n388 = Index Array(array=w1220, index=5) -> (element=w1218:dbl)
                          n389 = To Unsigned Word Integer(number=w1218) -> (unsigned 16bit integer=w1217:u16)
                          n390 = property on="Shutter Mode" class="Ring (strict)"("Val(Sgnl)"=w1217) -> ()  [unwired: 2 in, 2 out]
                          n391 = Wait (ms)(milliseconds to wait=w1219) -> ()  [unwired: 1 out]
                        }
                        frame #7 {
                          n392 = for {
                            tunnel: w1225 -> [w1237] mode=indexing
                            tunnel: w1224 -> [w1234]
                            tunnel: [w1231] -> w1223
                            tunnel: [w1230] -> w1222
                            i -> [w1231]
                            stop <- w1226 stop-if-true
                            n393 = Match Pattern(string=w1237, regular expression="[a-z]+") -> (match substring=w1229:string, after substring=w1228:string)  [unwired: 1 in, 2 out]
                            n394 = call <vilib>:"Trim Whitespace.vi"("string"=w1228) -> ("trimmed string"=w1235:string)  [unwired: 1 in]
                            n395 = Concatenate Strings(w1229, w1228) -> (w1227:string)
                            n396 = case shown="\"neutron\"" w1229 {
                              tunnel: w1235 -> [_ w1249 w1268 w1283 w1290 w1308 w1326 w1355]
                              tunnel: [TRUE ("Top Coil") w1248 w1265 FALSE ("Top Coil") w1287 w1305 w1325 w1354] -> w1233
                              tunnel: w1231 -> [w1241 w1247 w1267 _ w1289 w1307 w1324 w1353]
                              tunnel: w1234 -> [w1240 w1246 w1266 _ w1288 w1306 w1323 w1352]
                              tunnel: [w1238 w1244 w1263 "" ("Error String") w1285 w1304 w1321 w1350] -> w1230
                              tunnel: w1227 -> [w1239 w1243 w1262 _ w1284 w1303 w1320 w1349]
                              frame "False", Default {
                                n397 = call "ErrorHandling.vi"("Bad Command"=w1239, "Line #"=w1241, "Script #"=w1240) -> ("Error String"=w1238:string)  [unwired: 8 in]
                              }
                              frame "data" {
                                n398 = case shown="\"False\", Default" w1249 {
                                tunnel: [FALSE ("DATA") TRUE ("DATA") FALSE ("DATA")] -> w1245
                                tunnel: [TRUE ("Top Coil") FALSE ("Top Coil") FALSE ("Top Coil")] -> w1248
                                tunnel: w1247 -> [w1252 _ _]
                                tunnel: w1246 -> [w1253 _ _]
                                tunnel: [w1251 "" ""] -> w1244
                                tunnel: w1243 -> [w1250 _ _]
                                frame "False", Default {
                                n399 = call "ErrorHandling.vi"("Bad Command"=w1250, "Line #"=w1252, "Script #"=w1253) -> ("Error String"=w1251:string)  [unwired: 8 in]
                                }
                                frame "on" {
                                }
                                frame "off" {
                                }
                                }
                                n400 = property on="DATA" class="Bool (strict)"("Val(Sgnl)"=w1245) -> ()  [unwired: 2 in, 2 out]
                              }
                              frame "pulse" {
                                n401 = case shown="\"False\", Default" w1268 {
                                tunnel: [FALSE ("Top Coil") TRUE ("Top Coil") w1279] -> w1264
                                tunnel: [TRUE FALSE w1279] -> w1265
                                tunnel: w1267 -> [w1272 _ _]
                                tunnel: w1266 -> [w1271 _ _]
                                tunnel: [w1270 "" ("Error String") ""] -> w1263
                                tunnel: w1262 -> [w1269 _ _]
                                frame "False", Default {
                                n402 = call "ErrorHandling.vi"("Bad Command"=w1269, "Line #"=w1272, "Script #"=w1271) -> ("Error String"=w1270:string)  [unwired: 8 in]
                                }
                                frame "on" {
                                }
                                frame "off" {
                                w1279 = FALSE ("Top Coil")
                                }
                                }
                                n403 = property on="RUN/STOP" class="Bool (strict)"("Val(Sgnl)"=w1264) -> ()  [unwired: 2 in, 2 out]
                              }
                              frame "wait" {
                                n404 = Decimal String To Number(string=w1283) -> (number=w1282:i32)  [unwired: 2 in, 1 out]
                                n405 = Wait (ms)(milliseconds to wait=w1282) -> ()  [unwired: 1 out]
                              }
                              frame "neutron" {
                                n406 = case shown="\"False\", Default" w1290 {
                                tunnel: w1289 -> [w1296 _ _]
                                tunnel: w1288 -> [w1295 _ _]
                                tunnel: [TRUE ("Top Coil") FALSE ("Top Coil") w1301] -> w1287
                                tunnel: [FALSE ("Neutron Shutter") TRUE ("Neutron Shutter") w1301] -> w1286
                                tunnel: [w1292 "" ""] -> w1285
                                tunnel: w1284 -> [w1291 _ _]
                                frame "False", Default {
                                n407 = call "ErrorHandling.vi"("Bad Command"=w1291, "Line #"=w1296, "Script #"=w1295) -> ("Error String"=w1292:string)  [unwired: 8 in]
                                }
                                frame "on" {
                                }
                                frame "off" {
                                w1301 = FALSE ("Neutron Shutter")
                                }
                                }
                                n408 = property on="Neutron Shutter" class="Bool (strict)"("Val(Sgnl)"=w1286) -> ()  [unwired: 2 in, 2 out]
                              }
                              frame "shutter" {
                                n409 = case shown="\"off\"" w1308 {
                                tunnel: w1307 -> [w1314 _ _]
                                tunnel: w1306 -> [w1313 _ _]
                                tunnel: [TRUE ("Top Coil") FALSE ("Top Coil") w1319] -> w1305
                                tunnel: [FALSE ("Neutron Shutter") TRUE ("Neutron Shutter") w1319] -> w1302
                                tunnel: [w1310 "" ""] -> w1304
                                tunnel: w1303 -> [w1309 _ _]
                                frame "False", Default {
                                n410 = call "ErrorHandling.vi"("Bad Command"=w1309, "Line #"=w1314, "Script #"=w1313) -> ("Error String"=w1310:string)  [unwired: 8 in]
                                }
                                frame "on" {
                                }
                                frame "off" {
                                w1319 = FALSE ("Neutron Shutter")
                                }
                                }
                                n411 = property on="Enable" class="Bool (strict)"("Val(Sgnl)"=w1302) -> ()  [unwired: 2 in, 2 out]
                              }
                              frame "coila" {
                                n412 = case shown="\"False\", Default" w1326 {
                                selector: w1326 -> [w1333 _]
                                tunnel: [w1335 w1348] -> w1322
                                tunnel: [w1334 w1348] -> w1325
                                tunnel: w1324 -> [w1330 _]
                                tunnel: w1323 -> [w1329 _]
                                tunnel: [w1328 ""] -> w1321
                                tunnel: w1320 -> [w1327 _]
                                frame "False", Default {
                                n413 = Match Pattern(string=w1333, regular expression="[^0-9.]") -> (offset past match=w1331:i32)  [unwired: 1 in, 3 out]
                                n414 = case shown="-1" w1331 {
                                tunnel: [FALSE ("Top Coil") TRUE ("Top Coil")] -> w1335
                                tunnel: [TRUE FALSE] -> w1334
                                tunnel: w1333 -> [_ w1344]
                                tunnel: w1330 -> [w1339 _]
                                tunnel: w1329 -> [w1338 _]
                                tunnel: [w1337 ""] -> w1328
                                tunnel: w1327 -> [w1336 _]
                                frame 0, Default {
                                n415 = call "ErrorHandling.vi"("Bad Command"=w1336, "Line #"=w1339, "Script #"=w1338) -> ("Error String"=w1337:string)  [unwired: 8 in]
                                }
                                frame -1 {
                                n416 = Fract/Exp String To Number(string=w1344) -> (number=w1343:dbl)  [unwired: 3 in, 1 out]
                                n417 = property on="Top Coil (mA)" class="DigNum (strict)"("Val(Sgnl)"=w1343) -> ()  [unwired: 2 in, 2 out]
                                }
                                }
                                }
                                frame "off" {
                                w1348 = FALSE ("Top Coil")
                                }
                                }
                                n418 = property on="Top Coil" class="Bool (strict)"("Val(Sgnl)"=w1322) -> ()  [unwired: 2 in, 2 out]
                              }
                              frame "coilb" {
                                n419 = case shown="\"off\"" w1355 {
                                selector: w1355 -> [w1362 _]
                                tunnel: [w1361 w1377] -> w1351
                                tunnel: [w1360 w1377] -> w1354
                                tunnel: w1353 -> [w1359 _]
                                tunnel: w1352 -> [w1358 _]
                                tunnel: [w1357 "" ("Error String")] -> w1350
                                tunnel: w1349 -> [w1356 _]
                                frame "False", Default {
                                n420 = Match Pattern(string=w1362, regular expression="[^0-9.]") -> (offset past match=w1363:i32)  [unwired: 1 in, 3 out]
                                n421 = case shown="-1" w1363 {
                                tunnel: w1362 -> [_ w1375]
                                tunnel: [FALSE TRUE] -> w1361
                                tunnel: [TRUE FALSE] -> w1360
                                tunnel: w1359 -> [w1368 _]
                                tunnel: w1358 -> [w1367 _]
                                tunnel: [w1366 ""] -> w1357
                                tunnel: w1356 -> [w1365 _]
                                frame 0, Default {
                                n422 = call "ErrorHandling.vi"("Bad Command"=w1365, "Line #"=w1368, "Script #"=w1367) -> ("Error String"=w1366:string)  [unwired: 8 in]
                                }
                                frame -1 {
                                n423 = Fract/Exp String To Number(string=w1375) -> (number=w1372:dbl)  [unwired: 3 in, 1 out]
                                n424 = property on="Bottom Coil (mA)" class="DigNum (strict)"("Val(Sgnl)"=w1372) -> ()  [unwired: 2 in, 2 out]
                                }
                                }
                                }
                                frame "off" {
                                w1377 = FALSE
                                }
                                }
                                n425 = property on="Bottom Coil" class="Bool (strict)"("Val(Sgnl)"=w1351) -> ()  [unwired: 2 in, 2 out]
                              }
                            }
                            n426 = local read "Kill Switch"() -> (w1232:bool)
                            n427 = Or(x=w1233, y=w1232) -> (x .or. y?=w1226:bool)
                          }
                        }
                        frame #8 {
                          n428 = Decrement(x=w1392) -> (x-1=w1391:i32)
                          n429 = Equal?(x=w1393, y=w1391) -> (x = y?=w1381:bool)
                          n430 = local read "Error"() -> (w1378:bool)
                          n431 = Not(x=w1378) -> (.not. x?=w1379:bool)
                          n432 = And(x=w1381, y=w1379) -> (x .and. y?=w1380:bool)
                          n433 = case shown="False" w1380 {
                            tunnel: w1382 -> [w1405 w1412]
                            tunnel: [w1404 w1419] -> w1390
                            tunnel: w1389 -> [w1395 _]
                            tunnel: [w1399 w1413] -> w1388
                            tunnel: w1378 -> [_ _]
                            frame False {
                              w1398 = FALSE ("Value (Signaling)")
                              n434 = Equal?(x="", y=w1395) -> (x = y?=w1396:bool)
                              n435 = case shown="True" w1396 {
                                tunnel: w1395 -> [w1408 _]
                                tunnel: [w1408 "Temperature Warning!"] -> w1394
                                frame False {
                                }
                                frame True {
                                }
                              }
                              n436 = property on="Top Coil" class="Bool (strict)"("Val(Sgnl)"=w1398) -> ()  [unwired: 2 in, 2 out]
                              n437 = property on="Bottom Coil" class="Bool (strict)"("Val(Sgnl)"=w1398) -> ()  [unwired: 2 in, 2 out]
                              n438 = property on="SCRIPTING" class="Bool (strict)"("Val(Sgnl)"=w1398) -> ()  [unwired: 2 in, 2 out]
                              n439 = Number To Decimal String(number=w1405) -> (decimal integer string=w1402:string)  [unwired: 1 in]
                              n440 = property on="Neutron Shutter" class="Bool (strict)"("Val(Sgnl)"=w1398) -> ()  [unwired: 2 in, 2 out]
                              n441 = property on="DATA" class="Bool (strict)"("Val(Sgnl)"=w1398) -> ()  [unwired: 2 in, 2 out]
                              n442 = property on="RUN/STOP" class="Bool (strict)"("Val(Sgnl)"=w1398) -> ()  [unwired: 2 in, 2 out]
                              n443 = Concatenate Strings("Script" ("string"), w1402, " failed!" ("string"), "\r\n", w1394) -> (w1399:string)
                              n444 = property on="Enable" class="Bool (strict)"("Val(Sgnl)"=w1398) -> ()  [unwired: 2 in, 2 out]
                              n445 = Bundle(FALSE, 1017, w1399) -> (w1404:errorcluster)  [unwired: 1 in]
                            }
                            frame True {
                              n446 = Number To Decimal String(number=w1412) -> (decimal integer string=w1415:string)  [unwired: 1 in]
                              n447 = Less?(x=w1412, y="Script\nEnd") -> (x < y?=w1410:bool)
                              n448 = case shown="False" w1410 {
                                tunnel: w1412 -> [_ w1422]
                                frame False {
                                n449 = property on="SCRIPTING" class="Bool (strict)"("Val(Sgnl)"=FALSE ("Value (Signaling)")) -> ()  [unwired: 2 in, 2 out]
                                }
                                frame True {
                                n450 = Increment(x=w1422) -> (x+1=w1423:i32)
                                n451 = property on="Script\n#" class="DigNum (strict)"("Val(Sgnl)"=w1423) -> ()  [unwired: 2 in, 2 out]
                                n452 = Wait (ms)(milliseconds to wait=u32 5000) -> ()  [unwired: 1 out]
                                }
                              }
                              n453 = Concatenate Strings("Script" ("string"), w1415, " successful!" ("string")) -> (w1413:string)
                              n454 = Bundle(FALSE, 0, w1413) -> (w1419:errorcluster)  [unwired: 1 in]
                            }
                          }
                          "Scripting Error" <- w1390
                          n455 = local read "Timestamp"() -> (w1383:string)
                          n456 = call "WriteResults_Script.vi"("Timestamp"=w1383, "error in"=w1386, "Result"=w1388, "refnum in"=w1387) -> ("error out"=w1384:errorcluster, "refnum out"=w1385:refnum<file>)  [unwired: 6 in]
                        }
                      }
                      n457 = Array Size(array=w1182) -> (size(s)=w1181:i32)
                    }
                  }
                  n458 = flat-sequence {
                    tunnel: w1138 -> [w1149]
                    tunnel: [w1149] -> w1137
                    tunnel: [w1148] -> w1136
                    frame #0 {
                      n459 = local read "SCRIPTING"() -> (w1150:bool)
                      n460 = local read "Kill Switch"() -> (w1147:bool)
                      n461 = Not(x=w1150) -> (.not. x?=w1151:bool)
                      n462 = Or(x=w1151, y=w1147) -> (x .or. y?=w1148:bool)
                    }
                  }
                }
              }
            }
          }
        }
      }
      event "Fill": Value Change {
        n463 = event-data() -> ("NewVal"=w1432:bool)  [unwired: 1 in]
        n464 = case shown="True" w1432 {
          tunnel: w1430 -> [w1439 w1466]
          tunnel: w1431 -> [w1438 w1465]
          tunnel: [w1437 w1464] -> w1426
          tunnel: [w1436 w1463] -> w1427
          tunnel: w1429 -> [w1435 w1454]
          tunnel: [w1435 w1454] -> w1428
          frame False {
            n465 = flat-sequence {
              tunnel: w1439 -> [w1444]
              tunnel: w1438 -> [w1443]
              tunnel: [w1442] -> w1434
              tunnel: [w1441] -> w1433
              tunnel: [w1446] -> w1436
              tunnel: [w1447] -> w1437
              tunnel: w1434 -> [w1447]
              tunnel: w1433 -> [w1446]
              frame #0 {
                n466 = call "MFCSetpoint.vi"("MFC error in"=w1444, "MFC setpoint"=0.0, "MFC VISA in"=w1443) -> ("MFC error out"=w1441:errorcluster, "MFC VISA out"=w1442:refnum<visa-resource-name>)  [unwired: 7 in]
              }
              frame #1 {
                n467 = local write "3He Check"(TRUE ("3He Check")) -> ()
              }
            }
          }
          frame True {
            n468 = local read "Desired V2\nPressure (3He)"() -> (w1453:dbl)
            n469 = flat-sequence {
              tunnel: w1448 -> [w1468]
              tunnel: w1456 -> [w1469]
              tunnel: w1465 -> [w1470]
              tunnel: w1466 -> [w1471]
              tunnel: [w1471] -> w1452
              tunnel: [w1470] -> w1451
              tunnel: [w1469] -> w1450
              tunnel: [w1468] -> w1449
              tunnel: [w1475] -> w1462
              tunnel: [w1474] -> w1461
              tunnel: [w1472] -> w1458
              tunnel: w1452 -> [w1477]
              tunnel: w1451 -> [w1476]
              tunnel: w1450 -> [w1473]
              tunnel: w1449 -> [w1472]
              tunnel: w1462 -> [w1481]
              tunnel: w1461 -> [w1480]
              tunnel: [w1481] -> w1460
              tunnel: [w1480] -> w1459
              tunnel: w1458 -> [w1479]
              tunnel: w1455 -> [w1478]
              tunnel: [w1496] -> w1463
              tunnel: [w1497] -> w1464
              tunnel: w1460 -> [w1497]
              tunnel: w1459 -> [w1496]
              frame #0 {
                n470 = local write "3He Check"(FALSE ("3He Check")) -> ()
              }
              frame #1 {
                n471 = call "MFCSetpoint.vi"("MFC error in"=w1477, "MFC setpoint"=w1473, "MFC VISA in"=w1476) -> ("MFC error out"=w1474:errorcluster, "MFC VISA out"=w1475:refnum<visa-resource-name>)  [unwired: 7 in]
              }
              frame #2 {
                n472 = while {
                  tunnel: w1479 -> [w1494]
                  tunnel: w1478 -> [w1487]
                  i -> [w1490]
                  stop <- w1484 stop-if-true
                  n473 = local read "3He Pressure (Torr)"() -> (w1486:string)
                  n474 = Fract/Exp String To Number(string=w1486) -> (number=w1485:dbl)  [unwired: 3 in, 1 out]
                  n475 = Greater?(x=w1485, y=w1494) -> (0:w1493:bool)
                  n476 = Multiply(x=w1490, y=0.01) -> (x*y=w1489:dbl)
                  n477 = local read "Kill Switch"() -> (w1482:bool)
                  n478 = Greater?(x=w1489, y=w1487) -> (0:w1491:bool)
                  n479 = Or(x=w1491, y=w1493) -> (x .or. y?=w1483:bool)
                  n480 = Or(x=w1482, y=w1483) -> (x .or. y?=w1484:bool)
                  n481 = Wait (ms)(milliseconds to wait=u32 10) -> ()  [unwired: 1 out]
                }
              }
              frame #3 {
                n482 = property on="Fill" class="Bool (strict)"("Val(Sgnl)"=FALSE ("Value (Signaling)")) -> ()  [unwired: 2 in, 2 out]
              }
            }
            n483 = Add(x=w1454, y=w1453) -> (x+y=w1448:dbl)
            n484 = local read "Fill Time (s)"() -> (w1457:u32)
            n485 = call "MFCSettingCalc.vi"("Fill Time (s)"=w1457, "SetPoint"=w1453) -> ("Time (s)"=w1455:dbl, "MFC Setting"=w1456:dbl)  [unwired: 8 in]
          }
        }
      }
      event "Tare": Value Change {
        n486 = event-data() -> ("NewVal"=w1504:bool)  [unwired: 1 in]
        n487 = case shown="False" w1504 {
          tunnel: w1501 -> [w1505 _]
          tunnel: [w1505 w1506] -> w1500
          frame False {
          }
          frame True {
            n488 = local read "3He Pressure (Torr)"() -> (w1507:string)
            n489 = Fract/Exp String To Number(string=w1507) -> (number=w1506:dbl)  [unwired: 3 in, 1 out]
            n490 = local write "Tare"(FALSE ("Tare")) -> ()
          }
        }
      }
      event Timeout {
        n491 = event-data() -> ()  [unwired: 1 in, 3 out]
      }
    }
    n492 = local read "Kill Switch"() -> (w915:bool)
    n493 = And(x=w915, y="3He Check") -> (x .and. y?=w917:bool)
  }
  n494 = while {
    stop <- w1515 stop-if-true
    n495 = event shown="[0] Timeout" {
      selector: _ -> [_ _ _]
      dyn-events: _ -> [_ _ _]
      timeout: 500 -> [_ _ _]
      event Timeout {
        n496 = event-data() -> ()  [unwired: 1 in, 3 out]
      }
      event "COOLDOWN": Value Change {
        n497 = event-data() -> ("NewVal"=w1516:bool)  [unwired: 1 in, 5 out]
        n498 = case shown="True" w1516 {
          frame False {
          }
          frame True {
            n499 = flat-sequence {
              frame #0 {
                n500 = property on="Percent Open" class="DigNum (strict)"("Val(Sgnl)"=100 ("Percent Open")) -> ()  [unwired: 2 in, 2 out]
              }
              frame #1 {
                n501 = while {
                  i -> [w1521]
                  stop <- w1518 stop-if-true
                  n502 = Greater Than 0?(x=w1521) -> (x > 0?=w1520:bool)
                  n503 = case shown="True" w1520 {
                    tunnel: [FALSE ("Motor free") w1523] -> w1518
                    frame False {
                    }
                    frame True {
                      n504 = local read "Motor free"() -> (w1523:bool)
                    }
                  }
                  n505 = Wait (ms)(milliseconds to wait=u32 50) -> ()  [unwired: 1 out]
                }
              }
              frame #2 {
                n506 = property on="Sample Space Pump" class="Bool (strict)"("Val(Sgnl)"=FALSE ("Sample Space Pump")) -> ()  [unwired: 2 in, 2 out]
                n507 = Wait (ms)(milliseconds to wait=u32 250) -> ()  [unwired: 1 out]
              }
              frame #3 {
                n508 = property on="Siphon Pump" class="Bool (strict)"("Val(Sgnl)"=TRUE ("Siphon Pump")) -> ()  [unwired: 2 in, 2 out]
                n509 = Wait (ms)(milliseconds to wait=u32 250) -> ()  [unwired: 1 out]
              }
              frame #4 {
                n510 = while {
                  stop <- w1531 stop-if-true
                  n511 = local read "Kill Switch"() -> (w1534:bool)
                  n512 = local read "COOLDOWN"() -> (w1529:bool)
                  n513 = property on="Cryostat (K)" class="DigNum (strict)"() -> ("Value"=w1536:dbl)  [unwired: 2 in, 2 out]
                  n514 = Not(x=w1529) -> (.not. x?=w1528:bool)
                  n515 = Less?(x=w1536, y=3.8) -> (x < y?=w1533:bool)
                  n516 = Or(x=w1534, y=w1533) -> (x .or. y?=w1530:bool)
                  n517 = Or(x=w1530, y=w1528) -> (x .or. y?=w1531:bool)
                  n518 = Wait (ms)(milliseconds to wait=u32 1000) -> ()  [unwired: 1 out]
                }
              }
              frame #5 {
                n519 = while {
                  i -> [w1539]
                  stop <- w1538 stop-if-true
                  n520 = local read "COOLDOWN"() -> (w1544:bool)
                  n521 = local read "Kill Switch"() -> (w1541:bool)
                  n522 = Greater?(x=w1539, y="Time (s)") -> (0:w1540:bool)
                  n523 = Wait (ms)(milliseconds to wait=u32 1000) -> ()  [unwired: 1 out]
                  n524 = Not(x=w1544) -> (.not. x?=w1543:bool)
                  n525 = Or(x=w1540, y=w1541) -> (x .or. y?=w1542:bool)
                  n526 = Or(x=w1542, y=w1543) -> (x .or. y?=w1538:bool)
                }
              }
              frame #6 {
                n527 = property on="Percent Open" class="DigNum (strict)"("Val(Sgnl)"=0 ("Percent Open")) -> ()  [unwired: 2 in, 2 out]
              }
              frame #7 {
                n528 = while {
                  i -> [w1550]
                  stop <- w1547 stop-if-true
                  n529 = Greater Than 0?(x=w1550) -> (x > 0?=w1549:bool)
                  n530 = case shown="True" w1549 {
                    tunnel: [FALSE ("Motor free") w1552] -> w1547
                    frame False {
                    }
                    frame True {
                      n531 = local read "Motor free"() -> (w1552:bool)
                    }
                  }
                  n532 = Wait (ms)(milliseconds to wait=u32 50) -> ()  [unwired: 1 out]
                }
              }
              frame #8 {
                n533 = property on="Sample Space Pump" class="Bool (strict)"("Val(Sgnl)"=TRUE ("Sample Space Pump")) -> ()  [unwired: 2 in, 2 out]
                n534 = Wait (ms)(milliseconds to wait=u32 250) -> ()  [unwired: 1 out]
              }
              frame #9 {
                n535 = property on="Siphon Pump" class="Bool (strict)"("Val(Sgnl)"=FALSE ("Siphon Pump")) -> ()  [unwired: 2 in, 2 out]
                n536 = Wait (ms)(milliseconds to wait=u32 250) -> ()  [unwired: 1 out]
              }
              frame #10 {
                n537 = property on="COOLDOWN" class="Bool (strict)"("Val(Sgnl)"=FALSE ("COOLDOWN")) -> ()  [unwired: 2 in, 2 out]
              }
            }
          }
        }
      }
      event "REFILL": Value Change {
        n538 = event-data() -> ("NewVal"=w1558:bool)  [unwired: 1 in, 5 out]
        n539 = case shown="True" w1558 {
          frame False {
          }
          frame True {
            n540 = flat-sequence {
              frame #0 {
                n541 = property on="Percent Open" class="DigNum (strict)"("Val(Sgnl)"=100 ("Percent Open")) -> ()  [unwired: 2 in, 2 out]
              }
              frame #1 {
                n542 = while {
                  i -> [w1563]
                  stop <- w1560 stop-if-true
                  n543 = Greater Than 0?(x=w1563) -> (x > 0?=w1562:bool)
                  n544 = case shown="True" w1562 {
                    tunnel: [FALSE ("Motor free") w1565] -> w1560
                    frame False {
                    }
                    frame True {
                      n545 = local read "Motor free"() -> (w1565:bool)
                    }
                  }
                  n546 = Wait (ms)(milliseconds to wait=u32 50) -> ()  [unwired: 1 out]
                }
              }
              frame #2 {
                n547 = property on="Sample Space Pump" class="Bool (strict)"("Val(Sgnl)"=FALSE ("Sample Space Pump")) -> ()  [unwired: 2 in, 2 out]
                n548 = Wait (ms)(milliseconds to wait=u32 100) -> ()  [unwired: 1 out]
              }
              frame #3 {
                n549 = property on="Siphon Pump" class="Bool (strict)"("Val(Sgnl)"=TRUE ("Siphon Pump")) -> ()  [unwired: 2 in, 2 out]
                n550 = Wait (ms)(milliseconds to wait=u32 100) -> ()  [unwired: 1 out]
              }
              frame #4 {
                n551 = while {
                  stop <- w1572 stop-if-true
                  n552 = local read "High Level\n(Ohms)"() -> (w1571:dbl)
                  n553 = local read "AUTOFILL"() -> (w1577:bool)
                  n554 = local read "Kill Switch"() -> (w1574:bool)
                  n555 = Greater?(x=w1571, y="HL (Ohms)") -> (0:w1573:bool)
                  n556 = Wait (ms)(milliseconds to wait=u32 1000) -> ()  [unwired: 1 out]
                  n557 = Not(x=w1577) -> (.not. x?=w1576:bool)
                  n558 = Or(x=w1573, y=w1574) -> (x .or. y?=w1575:bool)
                  n559 = Or(x=w1575, y=w1576) -> (x .or. y?=w1572:bool)
                }
              }
              frame #5 {
                n560 = property on="Percent Open" class="DigNum (strict)"("Val(Sgnl)"=0 ("Percent Open")) -> ()  [unwired: 2 in, 2 out]
              }
              frame #6 {
                n561 = while {
                  i -> [w1583]
                  stop <- w1580 stop-if-true
                  n562 = Greater Than 0?(x=w1583) -> (x > 0?=w1582:bool)
                  n563 = case shown="True" w1582 {
                    tunnel: [FALSE ("Motor free") w1585] -> w1580
                    frame False {
                    }
                    frame True {
                      n564 = local read "Motor free"() -> (w1585:bool)
                    }
                  }
                  n565 = Wait (ms)(milliseconds to wait=u32 50) -> ()  [unwired: 1 out]
                }
              }
              frame #7 {
                n566 = property on="Sample Space Pump" class="Bool (strict)"("Val(Sgnl)"=TRUE ("Sample Space Pump")) -> ()  [unwired: 2 in, 2 out]
                n567 = Wait (ms)(milliseconds to wait=u32 100) -> ()  [unwired: 1 out]
              }
              frame #8 {
                n568 = property on="Siphon Pump" class="Bool (strict)"("Val(Sgnl)"=FALSE ("Siphon Pump")) -> ()  [unwired: 2 in, 2 out]
                n569 = Wait (ms)(milliseconds to wait=u32 100) -> ()  [unwired: 1 out]
              }
              frame #9 {
                n570 = property on="REFILL" class="Bool (strict)"("Val(Sgnl)"=FALSE ("COOLDOWN")) -> ()  [unwired: 2 in, 2 out]
              }
            }
          }
        }
      }
    }
    n571 = local read "Kill Switch"() -> (w1515:bool)
  }
  n572 = flat-sequence {
    tunnel: w31 -> [w1592]
    tunnel: [w1592] -> w30
    tunnel: [w1591] -> w29
    frame #0 {
      n573 = local read "LIGHTFIELD"() -> (w1591:bool)
    }
  }
  n574 = call "NeedleValveClose.vi"("error in (no error)"=w131, "VISA resource name"=w132) -> ("error out"=w55:errorcluster, "VISA resource name out"=w57:refnum<visa-resource-name>)  [unwired: 8 in]
  n575 = call "RelayControl.vi"("Neutron Shutter"=w79, "Error In"=w100, "Sample Space Pump"=w79, "Siphon Pump"=w79, "Relay In"=w98) -> ("Error Out"=w99:errorcluster, "Relay Out"=w97:refnum<visa-resource-name>)  [unwired: 5 in]
  n576 = flat-sequence {
    tunnel: [w1594] -> w26
    tunnel: w27 -> [w1594]
    tunnel: [w1593] -> w25
    frame #0 {
      n577 = local read "Enable"() -> (w1593:bool)
    }
  }
  n578 = flat-sequence {
    tunnel: [w1598] -> w93
    tunnel: [w1597] -> w94
    tunnel: w95 -> [w1596]
    tunnel: w96 -> [w1595]
    frame #0 {
      n579 = VISA Write(VISA resource name=w1596, write buffer=":PULSE0:STATE OFF\r\n" ("format string"), error in (no error)=w1595) -> (VISA resource name out=w1597:refnum<visa-resource-name>, error out=w1598:errorcluster)  [unwired: 1 out]
    }
  }
  n580 = VISA Close(VISA resource name=w97, error in (no error)=w99) -> (error out=w92:errorcluster)
  n581 = flat-sequence {
    tunnel: w55 -> [w1600]
    tunnel: [w1600] -> w58
    tunnel: [w1603] -> w56
    tunnel: w58 -> [w1603]
    frame #0 {
      n582 = Wait (ms)(milliseconds to wait=u32 3000) -> ()  [unwired: 1 out]
    }
    frame #1 {
      n583 = local write "Percent Open"(0 ("Percent Open")) -> ()
    }
  }
  n584 = case shown="True" w25 {
    tunnel: [w1605 w1609] -> w36
    tunnel: [w1604 w1608] -> w35
    tunnel: w34 -> [w1604 w1607]
    tunnel: w26 -> [w1605 w1606]
    frame False {
    }
    frame True {
      n585 = call "ToggleShutter.vi"("error in"=w1606, "VISA resource name"=w1607) -> ("error out"=w1609:errorcluster, "VISA resource name out"=w1608:refnum<visa-resource-name>)  [unwired: 8 in]
    }
  }
  n586 = VISA Close(VISA resource name=w15, error in (no error)=w16) -> (error out=→"Lakeshore218 Error":errorcluster)
  n587 = flat-sequence {
    tunnel: w79 -> [w1610]
    tunnel: [w1611] -> w91
    tunnel: w92 -> [w1611]
    frame #0 {
      n588 = local write "Siphon Pump"(w1610) -> ()
      n589 = local write "Sample Space Pump"(w1610) -> ()
      n590 = local write "Neutron Shutter"(w1610) -> ()
    }
  }
  n591 = Equal?(x=w29, y=TRUE) -> (x = y?=w37:bool)
  n592 = call <vilib>:"DAQmx Stop Task.vi"("task/channels in"=w49, "error in"=w48) -> ()  [unwired: 12 in, 2 out]
  n593 = call <vilib>:"DAQmx Stop Task.vi"("task/channels in"=w40, "error in"=w39) -> ()  [unwired: 12 in, 2 out]
  n594 = call <instrlib>:"Close.vi"("error in (no error)"=w146, "Mercury Reference"=w145) -> ("error out"=w111:errorcluster)  [unwired: 9 in]
  n595 = call <instrlib>:"Disconnect From Meter.vi"("Location of FieldMax2Lib.dll in"=w84, "Meter ID in"=w85) -> ()  [unwired: 7 in, 2 out]
  n596 = VISA Close(VISA resource name=w35, error in (no error)=w36) -> (error out=w33:errorcluster)
  n597 = call "KeithleyClose.vi"("Keithley Error In"=w107, "Node In"=w106, "KeithleyVISA In"=w105) -> ("Heater Error"=w104:errorcluster)  [unwired: 8 in]
  n598 = VISA Close(VISA resource name=w135, error in (no error)=w136) -> (error out=→"4He Gauge Error":errorcluster)
  n599 = call "3HeClose.vi"("error in (no error)"=w120, "VISA resource name"=w121) -> ("error out"=→"3He Gauge Error":errorcluster)  [unwired: 9 in]
  n600 = Not Equal?(x=refnum<file> refnum, y=w80) -> (x != y?=w82:bool)
  n601 = case shown="False" w37 {
    tunnel: w38 -> [w1612 w1616]
    tunnel: w30 -> [_ w1615]
    frame False {
      n602 = local write "LightField Error"(w1612) -> ()
    }
    frame True {
      n603 = call <userlib>:"Adv_Deregister_for_Callback.vi"("error in (no error)"=w1616, "LightField Automation in"=w1615) -> ("error out"=w1617:errorcluster, "LightField Automation out"=w1618:refnum<class "LightField Automation.lvclass">)  [unwired: 8 in]
      n604 = call <userlib>:"LFA_Close.vi"("error in (no error)"=w1617, "LightField Automation in"=w1618) -> ("error out"=w1614:errorcluster)  [unwired: 8 in, 1 out]
      n605 = flat-sequence {
        tunnel: w1614 -> [w1620]
        tunnel: [w1620] -> w1613
        frame #0 {
          n606 = local write "LIGHTFIELD"(FALSE ("LIGHTFIELD")) -> ()
        }
      }
      n607 = local write "LightField Error"(w1613) -> ()
    }
  }
  n608 = VISA Close(VISA resource name=w94, error in (no error)=w93) -> (error out=→"Pulse Generator Error":errorcluster)
  n609 = flat-sequence {
    tunnel: w104 -> [w1622]
    tunnel: [w1622] -> w103
    frame #0 {
      w1621 = FALSE ("Top Coil")
      n610 = local write "Top Coil"(w1621) -> ()
      n611 = local write "Bottom Coil"(w1621) -> ()
    }
  }
  n612 = VISA Close(VISA resource name=w57, error in (no error)=w56) -> (error out=w109:errorcluster)
  n613 = flat-sequence {
    tunnel: w33 -> [w1624]
    tunnel: [w1624] -> w32
    frame #0 {
      n614 = local write "Enable"(FALSE ("Enable")) -> ()
    }
  }
  n615 = case shown="True" w82 {
    tunnel: w81 -> [_ w1627]
    tunnel: w80 -> [_ w1626]
    frame False {
    }
    frame True {
      n616 = Close File(refnum=w1626, error in=w1627) -> (error out=w1625:errorcluster)  [unwired: 1 out]
      n617 = local write "File I/O Error"(w1625) -> ()
    }
  }
  n618 = flat-sequence {
    tunnel: w111 -> [w1634]
    tunnel: [w1634] -> w110
    tunnel: w109 -> [w1633]
    tunnel: [w1633] -> w108
    tunnel: [T2 {"status"=FALSE, "code"=0, "Description"=""} ("Scripting \nError")] -> w78
    tunnel: [w1631] -> w72
    tunnel: w73 -> [w1631]
    tunnel: w6 -> [w1629]
    tunnel: [w1629] -> w5
    tunnel: w3 -> [w1628]
    tunnel: [w1628] -> _
    frame #0 {
      w1630 = FALSE ("Kill Switch")
      n619 = local write "Kill Switch"(w1630) -> ()
      n620 = local write "READY"(w1630) -> ()
      n621 = local write "LIGHTFIELD"(w1630) -> ()
    }
  }
  n622 = VISA Close(VISA resource name=w7, error in (no error)=w8) -> (error out=w6:errorcluster)
  n623 = Close File(refnum=w75, error in=w74) -> (error out=w73:errorcluster)  [unwired: 1 out]
  n624 = local write "Scripting Error"(w78) -> ()
  "Temperature Error" <- w110
  "Heater Error" <- w103
  "Relay Errror" <- w91
  "Zaber Motor Error" <- w108
  "Log Error" <- w72
  "Shutter Error" <- w32
  "MFC Error Out" <- w5
